vi "resonant.calculation vi_MD.vi"() -> ()   [LabVIEW 2012]
uses:
  Custom Controls/display palette control.ctl
  Custom Controls/scan mode main settings tab.ctl
  <vilib>/Utility/miscctls.llb/LVMinMaxIncTypeDef.ctl
  <vilib>/Utility/miscctls.llb/LVOutOfRangeActionTypeDef.ctl
  Custom Controls/pixel resolution enum.ctl
  Custom Controls/experiment type.ctl
  Custom Controls/advanced settings inner tab CTL.ctl
  Custom Controls/MAIN Image panel reso tab Control type def.ctl
  Custom Controls/Histogram tab reso.ctl
  GFG/GFGnumericGet.vi
  GFG/GFGfpRefGet.vi
  GFG/GFGbooleanGet.vi
  GFG/GFGDisplayRefsGet.vi
  GFG/GFGImageRefsGet.vi
  GFG/GFG library.lvlib
panel:
  out "ready for flystart?":bool
  out "Numeric Control 2":i32
  in  "String":string
  out "Source VI":string
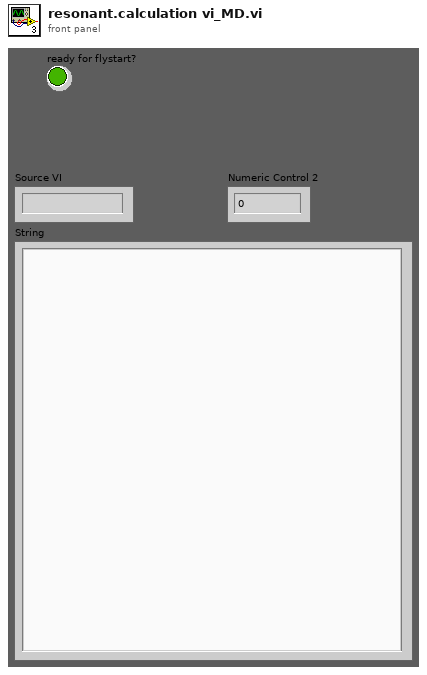
[diagram p1: front panel]
types:
  T1 = typedef "display palette control.ctl" = enum16{"standard", "high clipping red", "low clipping blue", "high and low clipping"}
  T2 = typedef "scan mode main settings tab.ctl" = enum32{"2D frame", "2D line scan", "general settings", "Z Stack", "piezo"}
  T3 = typedef "LVOutOfRangeActionTypeDef.ctl" = cluster{"Out of Range Action Minimum":u8, "Out of Range Action Maximum":u8, "Out of Range Action Increment":u8}
  T4 = typedef "LVMinMaxIncTypeDef.ctl" = cluster{"Minimum":dbl, "Maximum":dbl, "Increment":dbl}
  T5 = enum8{"Enabled", "Disabled", "Disabled and Grayed Out"}
  T6 = typedef "pixel resolution enum.ctl" = enum16{"   128 x 128", "   256 x 128", "   256 x 256", "   512 x  64", "   512 x 128", "   512 x 256", "   512 x 512", "  1024 x 512", "  1024 x 1024", "   arbitrary"}
  T7 = typedef "experiment type.ctl" = string
  T8 = enum32{"Page Enabled", "Page Disabled", "Page Disabled & Grayed"}
  T9 = typedef "advanced settings inner tab CTL.ctl" = enum32{"arb. frames", "AO", "AI", "channels", "trigger", "Zstack data"}
  T10 = typedef "MAIN Image panel reso tab Control type def.ctl" = enum32{"Channel 1", "Channel 2", "Channel 3", "Channel 4", "Channel 5", "all channels", "RGB overlay", "ROI", "arbitrary line scan"}
  T11 = typedef "Histogram tab reso.ctl" = enum32{"hist Ch 1", "hist Ch 4", "hist Ch 5", "hist Ch 3", "hist Ch 2"}
  T12 = cluster{"WaveformChartRef":refnum<vi>, "DigitalRef":refnum<vi>, "ArrayRef":refnum<vi>, "TabControlRef":refnum<vi>, "EnumRef":refnum<vi>, "RingRef":refnum<vi>, "BooleanRef":refnum<vi>, "KnobRef":refnum<vi>, "SlideRef":refnum<vi>, "PathRef":refnum<vi>, "StringRef":refnum<vi>, "ComboBox":refnum<vi>, "WaveformGraphRef":refnum<vi>}
  T13 = cluster{"Channel 1 small":refnum<vi>, "Channel 2 small":refnum<vi>, "Channel 3 small":refnum<vi>, "Channel 4 small":refnum<vi>, "Channel 1 large":refnum<vi>, "Channel 2 large":refnum<vi>, "Channel 3 large":refnum<vi>, "Channel 4 large":refnum<vi>, "RGB overlay":refnum<vi>, "ROI Image display":refnum<vi>, "arb line scan display":refnum<vi>, "Channel 5 large":refnum<vi>}
  T14 = typedef "IMAQ Image.ctl" = refnum<image>
  T15 = cluster{"Channel 1 small":T14, "Channel 2 small":T14, "Channel 3 small":T14, "Channel 4 small":T14, "Channel 1 large":T14, "Channel 2 large":T14, "Channel 3 large":T14, "Channel 4 large":T14, "RGB overlay":T14, "ROI Image display":T14, "arb line scan display":T14, "Channel 5 large":T14}
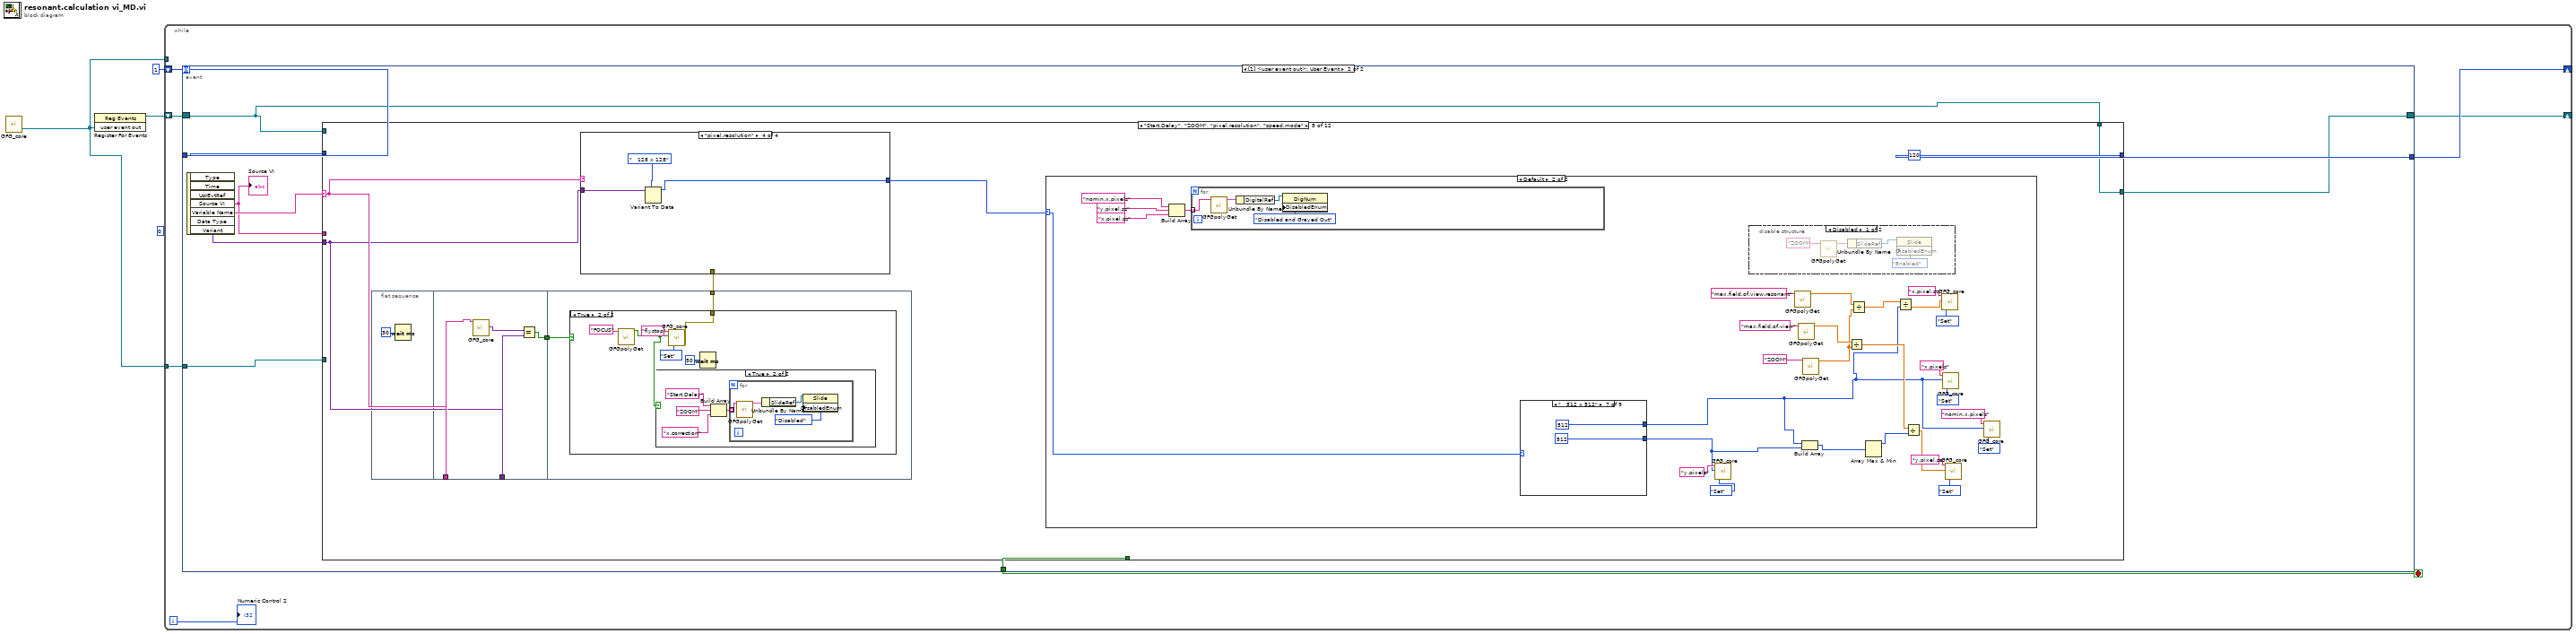
[diagram p0: block diagram]
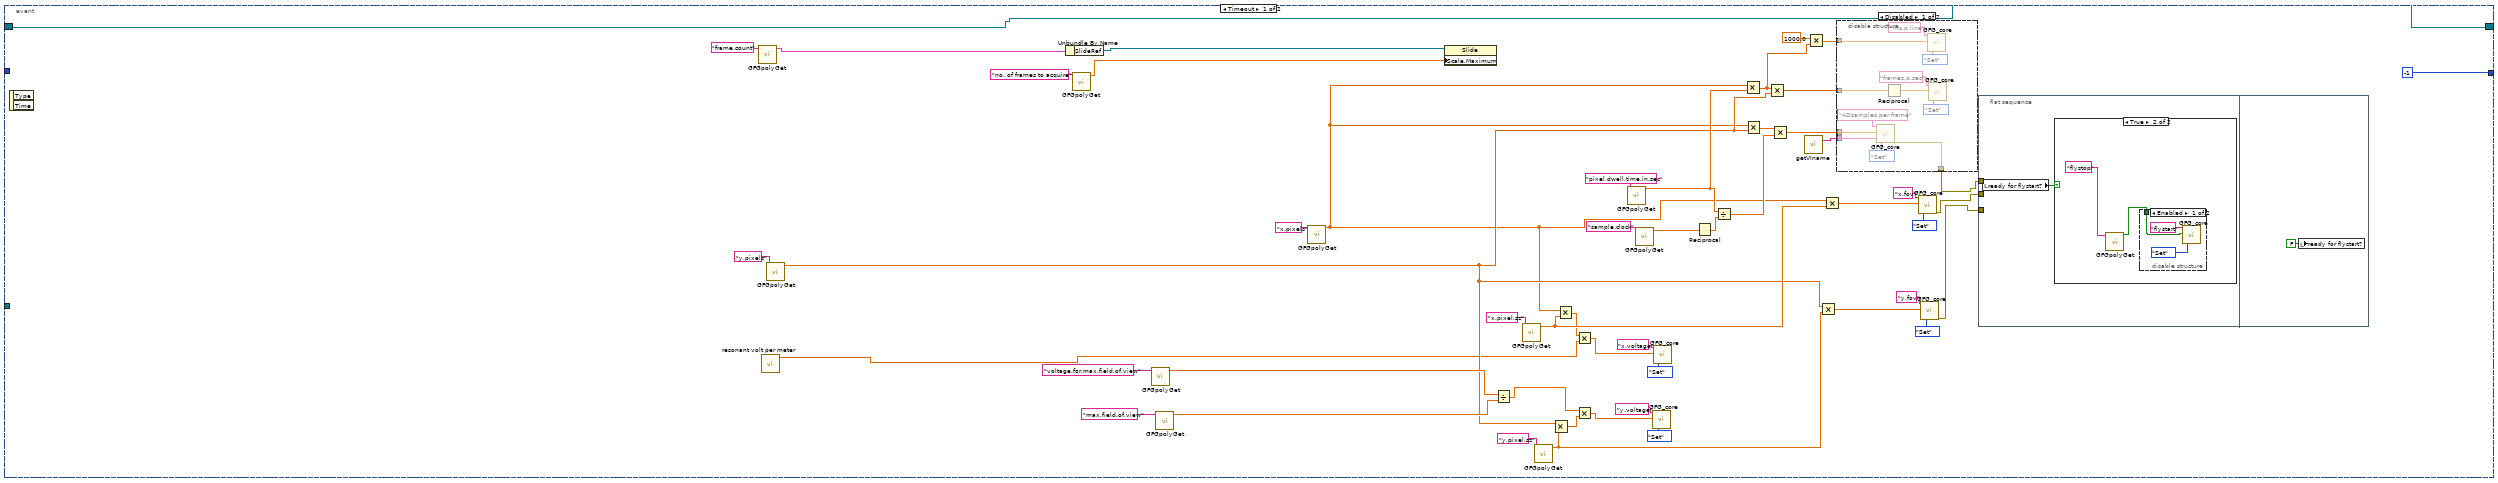
[diagram p2: hidden frame]
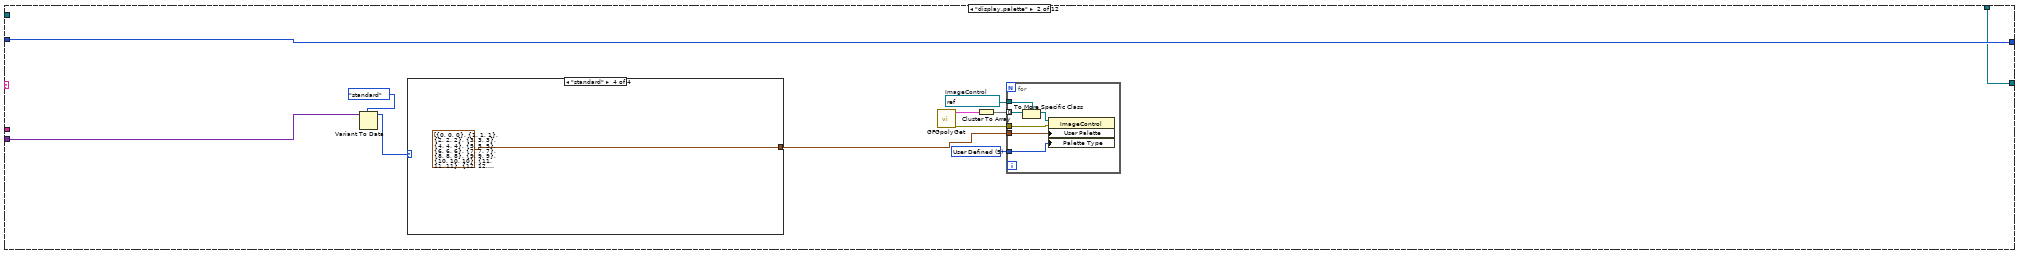
[diagram p7: hidden frame]
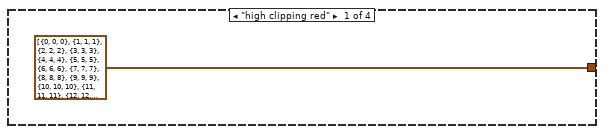
[diagram p8: hidden frame]
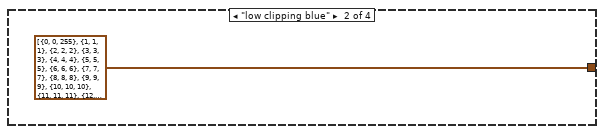
[diagram p9: hidden frame]
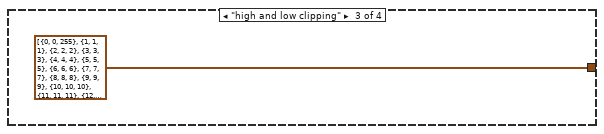
[diagram p10: hidden frame]
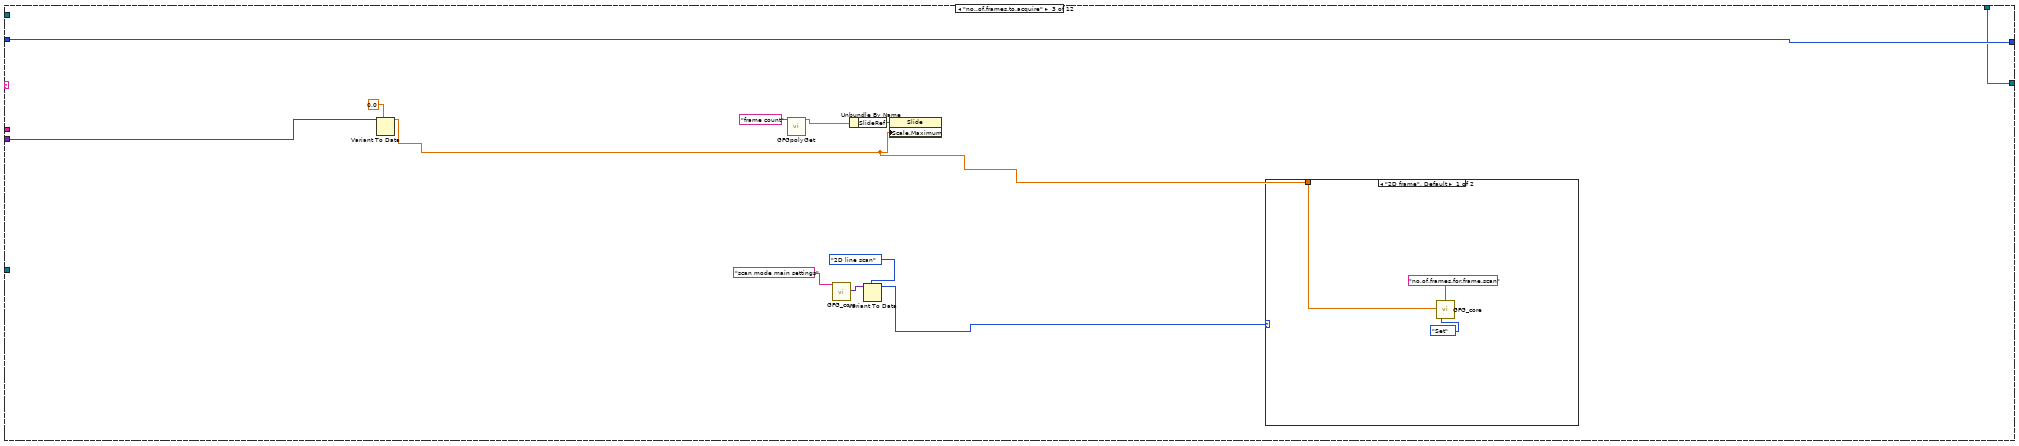
[diagram p11: hidden frame]
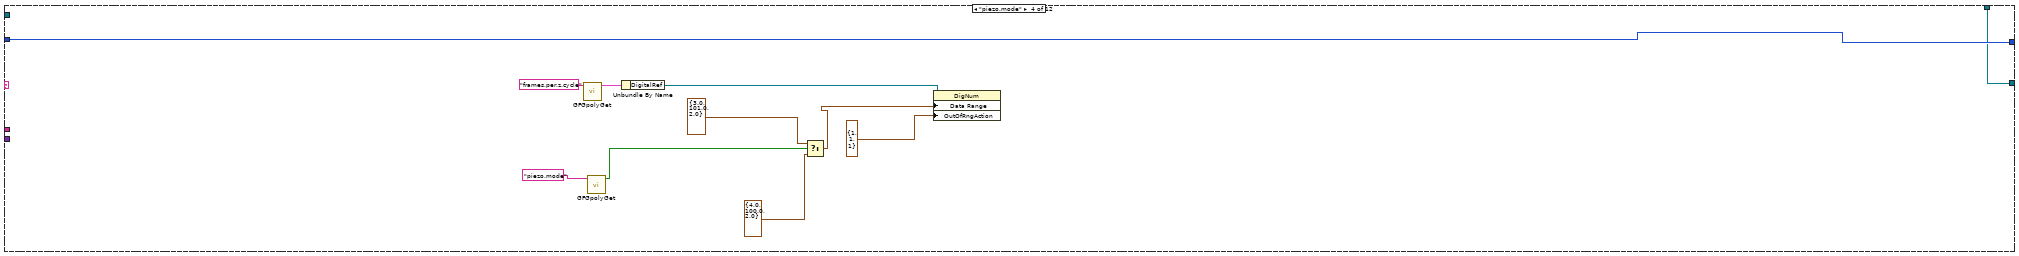
[diagram p13: hidden frame]
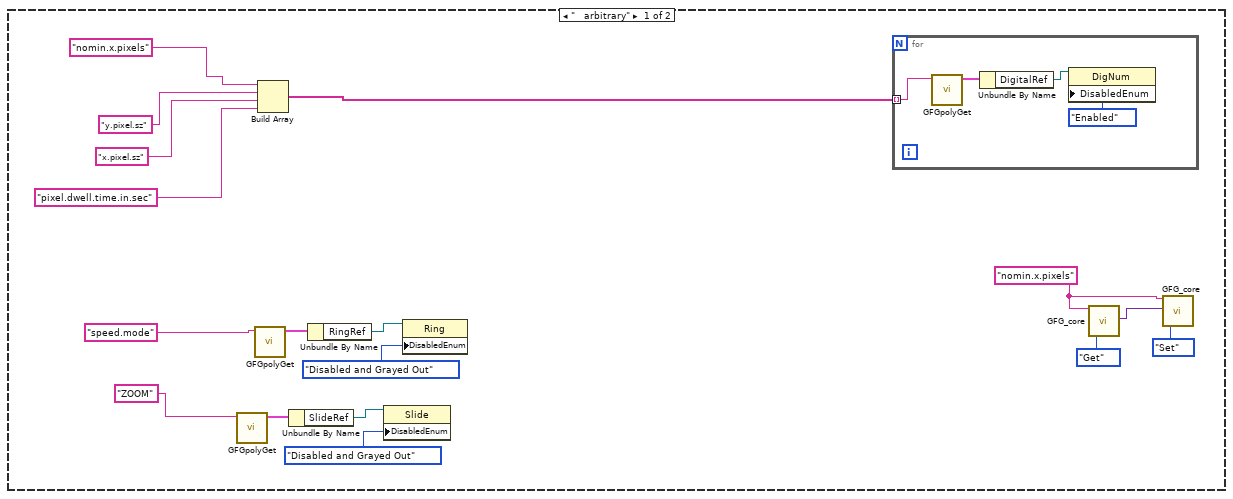
[diagram p16: hidden frame]
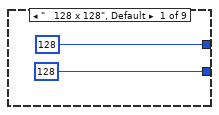
[diagram p18: hidden frame]
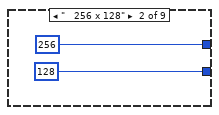
[diagram p19: hidden frame]
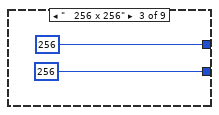
[diagram p20: hidden frame]
diagram:
  (unwired) 0
  n1 = call "GFG_core.vi"() -> ("user event out"=w1:refnum<user-event>)  [unwired: 13 in, 6 out]
  n2 = register-events(w1) -> (reference out=w3:refnum<event-registration>)  [unwired: 2 in, 1 out]
  n3 = while {
    shift-right: [w8] -> _
    shift-left: 1 -> [w7]
    tunnel: w1 -> [_]
    shift-right: [w4] -> _
    shift-left: w3 -> [w10]
    tunnel: w1 -> [w5]
    i -> [w6]
    stop <- w9 stop-if-true
    n4 = event shown="[1] <user event out>: User Event" {
      selector: w10 -> [w16 w82]
      dyn-events: [w16 w81] -> w4
      timeout: w7 -> [_ _]
      tunnel: [_ w88] -> w9
      tunnel: [-1 w86] -> w8
      tunnel: w7 -> [_ w85]
      tunnel: w5 -> [_ w83]
      event Timeout {
        n5 = event-data() -> ()  [unwired: 1 in, 2 out]
        n6 = call-poly "GFGpolyGet.vi"("Variable Name in"="frame.count") -> ("output cluster"=w20:T12)  [unwired: 9 in, 1 out]
        n7 = call "resonant volt per meter.vi"() -> ("volt/meter interpolated"=w15:dbl)  [unwired: 11 in]
        n8 = call-poly "GFGpolyGet.vi"("Variable Name in"="y.pixels") -> ("Numeric"=w22:dbl)  [unwired: 9 in, 1 out]
        n9 = Unbundle By Name(w20) -> ("SlideRef"=w19:refnum<vi>)
        n10 = call-poly "GFGpolyGet.vi"("Variable Name in"="no. of frames to acquire") -> ("Numeric"=w17:dbl)  [unwired: 9 in, 1 out]
        n11 = call-poly "GFGpolyGet.vi"("Variable Name in"="voltage.for.max.field.of.view") -> ("Numeric"=w41:dbl)  [unwired: 9 in, 1 out]
        n12 = call-poly "GFGpolyGet.vi"("Variable Name in"="max.field.of.view") -> ("Numeric"=w42:dbl)  [unwired: 9 in, 1 out]
        n13 = call-poly "GFGpolyGet.vi"("Variable Name in"="x.pixels") -> ("Numeric"=w11:dbl)  [unwired: 9 in, 1 out]
        n14 = property class="Slide"(reference=w19, "Scale.Maximum"=w17) -> ()  [unwired: 1 in, 2 out]
        n15 = Divide(x=w41, y=w42) -> (x/y=w40:dbl)
        n16 = call-poly "GFGpolyGet.vi"("Variable Name in"="x.pixel.sz") -> ("Numeric"=w33:dbl)  [unwired: 9 in, 1 out]
        n17 = call-poly "GFGpolyGet.vi"("Variable Name in"="y.pixel.sz") -> ("Numeric"=w31:dbl)  [unwired: 9 in, 1 out]
        n18 = Multiply(x=w22, y=w31) -> (x*y=w30:dbl)
        n19 = Multiply(x=w11, y=w33) -> (x*y=w32:dbl)
        n20 = Multiply(x=w32, y=w15) -> (x*y=w35:dbl)
        n21 = Multiply(x=w40, y=w30) -> (x*y=w34:dbl)
        n22 = call-poly "GFGpolyGet.vi"("Variable Name in"="pixel.dwell.time.in.sec") -> ("Numeric"=w26:dbl)  [unwired: 9 in, 1 out]
        n23 = call-poly "GFGpolyGet.vi"("Variable Name in"="sample.clock") -> ("Numeric"=w29:dbl)  [unwired: 9 in, 1 out]
        n24 = call "GFG_core.vi"("Variable Name in"="y.voltage", "Variant in"=w34, "Action"=enum16{"Init", "Set", "Get"}."Set") -> ()  [unwired: 10 in, 7 out]
        n25 = call "GFG_core.vi"("Variable Name in"="x.voltage", "Variant in"=w35, "Action"=enum16{"Init", "Set", "Get"}."Set") -> ()  [unwired: 10 in, 7 out]
        n26 = Reciprocal(x=w29) -> (1/x=w49:dbl)
        n27 = Divide(x=w26, y=w49) -> (x/y=w47:dbl)
        n28 = Multiply(x=w11, y=w26) -> (x*y=w25:dbl)
        n29 = Multiply(x=w11, y=w22) -> (x*y=w28:dbl)
        n30 = Multiply(x=w25, y=w22) -> (x*y=w27:dbl)
        n31 = Multiply(x=w28, y=w47) -> (x*y=w60:dbl)
        n32 = call "getVIname.vi"() -> ("VI name"=w59:string)  [unwired: 19 in]
        n33 = Multiply(x=1000.0, y=w25) -> (x*y=w23:dbl)
        n34 = Multiply(x=w22, y=w31) -> (x*y=w51:dbl)
        n35 = Multiply(x=w11, y=w33) -> (x*y=w54:dbl)
        n36 = disable-structure shown="Disabled" {
          disable-tunnel: w60 -> [w79 _]
          disable-tunnel: w59 -> [w77 _]
          disable-tunnel: [w76 _] -> w14
          disable-tunnel: w27 -> [w71 _]
          disable-tunnel: w23 -> [w69 _]
          frame Disabled {
            n37 = call "GFG_core.vi"("Variable Name in"="ADsamples.per.frame", "Variant in"=w79, "Source VI"=w77, "Action"=enum16{"Init", "Set", "Get"}."Set") -> ("error out"=w76:errorcluster)  [unwired: 9 in, 6 out]
            n38 = Reciprocal(x=w71) -> (1/x=w70:dbl)
            n39 = call "GFG_core.vi"("Variable Name in"="ms.p.line", "Variant in"=w69, "Action"=enum16{"Init", "Set", "Get"}."Set") -> ()  [unwired: 10 in, 7 out]
            n40 = call "GFG_core.vi"("Variable Name in"="frames.p.sec", "Variant in"=w70, "Action"=enum16{"Init", "Set", "Get"}."Set") -> ()  [unwired: 10 in, 7 out]
          }
          frame Enabled {
          }
        }
        n41 = call "GFG_core.vi"("Variable Name in"="x.fov", "Variant in"=w54, "Action"=enum16{"Init", "Set", "Get"}."Set") -> ("error out"=w13:errorcluster)  [unwired: 10 in, 6 out]
        n42 = call "GFG_core.vi"("Variable Name in"="y.fov", "Variant in"=w51, "Action"=enum16{"Init", "Set", "Get"}."Set") -> ("error out"=w12:errorcluster)  [unwired: 10 in, 6 out]
        n43 = flat-sequence {
          tunnel: w14 -> [_]
          tunnel: w13 -> [_]
          tunnel: w12 -> [_]
          frame #0 {
            n44 = local read "ready for flystart?"() -> (w62:bool)
            n45 = case shown="True" w62 {
              frame False {
              }
              frame True {
                n46 = call-poly "GFGpolyGet.vi"("Variable Name in"="flystop") -> ("Boolean"=w63:bool)  [unwired: 10 in]
                n47 = disable-structure shown="Enabled" {
                  disable-tunnel: w63 -> [w65 _]
                  frame Enabled {
                    n48 = call "GFG_core.vi"("Variable Name in"="flystart", "Variant in"=w65, "Action"=enum16{"Init", "Set", "Get"}."Set") -> ()  [unwired: 10 in, 7 out]
                  }
                  frame Disabled {
                  }
                }
              }
            }
          }
          frame #1 {
            n49 = local write "ready for flystart?"(FALSE ("ready for flystart?")) -> ()
          }
        }
      }
      event User Event {
        n50 = event-data() -> ("Source VI"=w84:string, "Variable Name"=w89:string, "Variant"=w87:variant)  [unwired: 1 in, 4 out]
        "Source VI" <- w84
        n51 = case shown="\"Start.Delay\", \"ZOOM\", \"pixel.resolution\", \"speed.mode\"" w89 {
          selector: w89 -> [_ _ _ _ w142 _ _ _ w342 _ _ _]
          tunnel: [_ _ _ _ _ _ _ _ _ _ _ TRUE] -> w88
          tunnel: w87 -> [_ w102 w121 _ w141 _ _ w296 _ w369 w399 _]
          tunnel: [w91 w99 w119 w138 120 w275 w283 w292 150 w366 w400 w402] -> w86
          tunnel: w85 -> [w91 w99 w119 w138 _ w275 w283 w293 _ w367 w400 w402]
          tunnel: w84 -> [_ _ _ _ _ _ _ _ _ _ _ _]
          tunnel: w82 -> [_ _ _ _ _ w274 _ _ _ _ _ _]
          tunnel: w83 -> [_ _ _ _ _ _ _ _ _ _ _ _]
          tunnel: [w90 w92 w113 w128 w143 w274 w284 w291 w343 w361 w380 w401] -> w81
          tunnel: w82 -> [w90 w92 w113 w128 w143 _ w284 w291 w343 w361 w380 w401]
          frame "False", Default {
          }
          frame "display.palette" {
            w94 = u32 5 items=["Grayscale", "Binary", "Gradient", "Rainbow", "Temperature", "User Defined"] ("Palette:Palette Type")
            w96 = refnum<vi> refnum  # ImageControl
            n52 = Variant To Data(type=display_palette_control."standard" ("display palette"), Variant=w102) -> (data=w100:T1)  [unwired: 1 in, 1 out]
            n53 = case shown="\"standard\"" w100 {
              tunnel: [cluster{"Red":u8, "Green":u8, "Blue":u8}[] [{"Red"=0, "Green"=0, "Blue"=0}, {"Red"=1, "Green"=1, "Blue"=1}, {"Red"=2, "Green"=2, "Blue"=2}, {"Red"=3, "Green"=3, "Blue"=3}, {"Red"=4, "Green"=4, "Blue"=4}, {"Red"=5, "Green"=5, "Blue"=5}, {"Red"=6, "Green"=6, "Blue"=6}, {"Red"=7, "Green"=7, "Blue"=7}, {"Red"=8, "Green"=8, "Blue"=8}, {"Red"=9, "Green"=9, "Blue"=9}, {"Red"=10, "Green"=10, "Blue"=10}, {"Red"=11, "Green"=11, "Blue"=11}, {"Red"=12, "Green"=12, "Blue"=12}, {"Red"=13, "Green"=13, "Blue"=13}, {"Red"=14, "Green"=14, "Blue"=14}, {"Red"=15, "Green"=15, "Blue"=15}, {"Red"=16, "Green"=16, "Blue"=16}, {"Red"=17, "Green"=17, "Blue"=17}, {"Red"=18, "Green"=18, "Blue"=18}, {"Red"=19, "Green"=19, "Blue"=19}, {"Red"=20, "Green"=20, "Blue"=20}, {"Red"=21, "Green"=21, "Blue"=21}, {"Red"=22, "Green"=22, "Blue"=22}, {"Red"=23, "Green"=23, "Blue"=23}, {"Red"=24, "Green"=24, "Blue"=24}, {"Red"=25, "Green"=25, "Blue"=25}, {"Red"=26, "Green"=26, "Blue"=26}, {"Red"=27, "Green"=27, "Blue"=27}, {"Red"=28, "Green"=28, "Blue"=28}, {"Red"=29, "Green"=29, "Blue"=29}, {"Red"=30, "Green"=30, "Blue"=30}, {"Red"=31, "Green"=31, "Blue"=31}, {"Red"=32, "Green"=32, "Blue"=32}, {"Red"=33, "Green"=33, "Blue"=33}, {"Red"=34, "Green"=34, "Blue"=34}, {"Red"=35, "Green"=35, "Blue"=35}, {"Red"=36, "Green"=36, "Blue"=36}, {"Red"=37, "Green"=37, "Blue"=37}, {"Red"=38, "Green"=38, "Blue"=38}, {"Red"=39, "Green"=39, "Blue"=39}, {"Red"=40, "Green"=40, "Blue"=40}, {"Red"=41, "Green"=41, "Blue"=41}, {"Red"=42, "Green"=42, "Blue"=42}, {"Red"=43, "Green"=43, "Blue"=43}, {"Red"=44, "Green"=44, "Blue"=44}, {"Red"=45, "Green"=45, "Blue"=45}, {"Red"=46, "Green"=46, "Blue"=46}, {"Red"=47, "Green"=47, "Blue"=47}, {"Red"=48, "Green"=48, "Blue"=48}, {"Red"=49, "Green"=49, "Blue"=49}, {"Red"=50, "Green"=50, "Blue"=50}, {"Red"=51, "Green"=51, "Blue"=51}, {"Red"=52, "Green"=52, "Blue"=52}, {"Red"=53, "Green"=53, "Blue"=53}, {"Red"=54, "Green"=54, "Blue"=54}, {"Red"=55, "Green"=55, "Blue"=55}, {"Red"=56, "Green"=56, "Blue"=56}, {"Red"=57, "Green"=57, "Blue"=57}, {"Red"=58, "Green"=58, "Blue"=58}, {"Red"=59, "Green"=59, "Blue"=59}, {"Red"=60, "Green"=60, "Blue"=60}, {"Red"=61, "Green"=61, "Blue"=61}, {"Red"=62, "Green"=62, "Blue"=62}, {"Red"=63, "Green"=63, "Blue"=63}, {"Red"=64, "Green"=64, "Blue"=64}, {"Red"=65, "Green"=65, "Blue"=65}, {"Red"=66, "Green"=66, "Blue"=66}, {"Red"=67, "Green"=67, "Blue"=67}, {"Red"=68, "Green"=68, "Blue"=68}, {"Red"=69, "Green"=69, "Blue"=69}, {"Red"=70, "Green"=70, "Blue"=70}, {"Red"=71, "Green"=71, "Blue"=71}, {"Red"=72, "Green"=72, "Blue"=72}, {"Red"=73, "Green"=73, "Blue"=73}, {"Red"=74, "Green"=74, "Blue"=74}, {"Red"=75, "Green"=75, "Blue"=75}, {"Red"=76, "Green"=76, "Blue"=76}, {"Red"=77, "Green"=77, "Blue"=77}, {"Red"=78, "Green"=78, "Blue"=78}, {"Red"=79, "Green"=79, "Blue"=79}, {"Red"=80, "Green"=80, "Blue"=80}, {"Red"=81, "Green"=81, "Blue"=81}, {"Red"=82, "Green"=82, "Blue"=82}, {"Red"=83, "Green"=83, "Blue"=83}, {"Red"=84, "Green"=84, "Blue"=84}, {"Red"=85, "Green"=85, "Blue"=85}, {"Red"=86, "Green"=86, "Blue"=86}, {"Red"=87, "Green"=87, "Blue"=87}, {"Red"=88, "Green"=88, "Blue"=88}, {"Red"=89, "Green"=89, "Blue"=89}, {"Red"=90, "Green"=90, "Blue"=90}, {"Red"=91, "Green"=91, "Blue"=91}, {"Red"=92, "Green"=92, "Blue"=92}, {"Red"=93, "Green"=93, "Blue"=93}, {"Red"=94, "Green"=94, "Blue"=94}, {"Red"=95, "Green"=95, "Blue"=95}, {"Red"=96, "Green"=96, "Blue"=96}, {"Red"=97, "Green"=97, "Blue"=97}, {"Red"=98, "Green"=98, "Blue"=98}, {"Red"=99, "Green"=99, "Blue"=99}, {"Red"=100, "Green"=100, "Blue"=100}, {"Red"=101, "Green"=101, "Blue"=101}, {"Red"=102, "Green"=102, "Blue"=102}, {"Red"=103, "Green"=103, "Blue"=103}, {"Red"=104, "Green"=104, "Blue"=104}, {"Red"=105, "Green"=105, "Blue"=105}, {"Red"=106, "Green"=106, "Blue"=106}, {"Red"=107, "Green"=107, "Blue"=107}, {"Red"=108, "Green"=108, "Blue"=108}, {"Red"=109, "Green"=109, "Blue"=109}, {"Red"=110, "Green"=110, "Blue"=110}, {"Red"=111, "Green"=111, "Blue"=111}, {"Red"=112, "Green"=112, "Blue"=112}, {"Red"=113, "Green"=113, "Blue"=113}, {"Red"=114, "Green"=114, "Blue"=114}, {"Red"=115, "Green"=115, "Blue"=115}, {"Red"=116, "Green"=116, "Blue"=116}, {"Red"=117, "Green"=117, "Blue"=117}, {"Red"=118, "Green"=118, "Blue"=118}, {"Red"=119, "Green"=119, "Blue"=119}, {"Red"=120, "Green"=120, "Blue"=120}, {"Red"=121, "Green"=121, "Blue"=121}, {"Red"=122, "Green"=122, "Blue"=122}, {"Red"=123, "Green"=123, "Blue"=123}, {"Red"=124, "Green"=124, "Blue"=124}, {"Red"=125, "Green"=125, "Blue"=125}, {"Red"=126, "Green"=126, "Blue"=126}, {"Red"=127, "Green"=127, "Blue"=127}, {"Red"=128, "Green"=128, "Blue"=128}, {"Red"=129, "Green"=129, "Blue"=129}, {"Red"=130, "Green"=130, "Blue"=130}, {"Red"=131, "Green"=131, "Blue"=131}, {"Red"=132, "Green"=132, "Blue"=132}, {"Red"=133, "Green"=133, "Blue"=133}, {"Red"=134, "Green"=134, "Blue"=134}, {"Red"=135, "Green"=135, "Blue"=135}, {"Red"=136, "Green"=136, "Blue"=136}, {"Red"=137, "Green"=137, "Blue"=137}, {"Red"=138, "Green"=138, "Blue"=138}, {"Red"=139, "Green"=139, "Blue"=139}, {"Red"=140, "Green"=140, "Blue"=140}, {"Red"=141, "Green"=141, "Blue"=141}, {"Red"=142, "Green"=142, "Blue"=142}, {"Red"=143, "Green"=143, "Blue"=143}, {"Red"=144, "Green"=144, "Blue"=144}, {"Red"=145, "Green"=145, "Blue"=145}, {"Red"=146, "Green"=146, "Blue"=146}, {"Red"=147, "Green"=147, "Blue"=147}, {"Red"=148, "Green"=148, "Blue"=148}, {"Red"=149, "Green"=149, "Blue"=149}, {"Red"=150, "Green"=150, "Blue"=150}, {"Red"=151, "Green"=151, "Blue"=151}, {"Red"=152, "Green"=152, "Blue"=152}, {"Red"=153, "Green"=153, "Blue"=153}, {"Red"=154, "Green"=154, "Blue"=154}, {"Red"=155, "Green"=155, "Blue"=155}, {"Red"=156, "Green"=156, "Blue"=156}, {"Red"=157, "Green"=157, "Blue"=157}, {"Red"=158, "Green"=158, "Blue"=158}, {"Red"=159, "Green"=159, "Blue"=159}, {"Red"=160, "Green"=160, "Blue"=160}, {"Red"=161, "Green"=161, "Blue"=161}, {"Red"=162, "Green"=162, "Blue"=162}, {"Red"=163, "Green"=163, "Blue"=163}, {"Red"=164, "Green"=164, "Blue"=164}, {"Red"=165, "Green"=165, "Blue"=165}, {"Red"=166, "Green"=166, "Blue"=166}, {"Red"=167, "Green"=167, "Blue"=167}, {"Red"=168, "Green"=168, "Blue"=168}, {"Red"=169, "Green"=169, "Blue"=169}, {"Red"=170, "Green"=170, "Blue"=170}, {"Red"=171, "Green"=171, "Blue"=171}, {"Red"=172, "Green"=172, "Blue"=172}, {"Red"=173, "Green"=173, "Blue"=173}, {"Red"=174, "Green"=174, "Blue"=174}, {"Red"=175, "Green"=175, "Blue"=175}, {"Red"=176, "Green"=176, "Blue"=176}, {"Red"=177, "Green"=177, "Blue"=177}, {"Red"=178, "Green"=178, "Blue"=178}, {"Red"=179, "Green"=179, "Blue"=179}, {"Red"=180, "Green"=180, "Blue"=180}, {"Red"=181, "Green"=181, "Blue"=181}, {"Red"=182, "Green"=182, "Blue"=182}, {"Red"=183, "Green"=183, "Blue"=183}, {"Red"=184, "Green"=184, "Blue"=184}, {"Red"=185, "Green"=185, "Blue"=185}, {"Red"=186, "Green"=186, "Blue"=186}, {"Red"=187, "Green"=187, "Blue"=187}, {"Red"=188, "Green"=188, "Blue"=188}, {"Red"=189, "Green"=189, "Blue"=189}, {"Red"=190, "Green"=190, "Blue"=190}, {"Red"=191, "Green"=191, "Blue"=191}, {"Red"=192, "Green"=192, "Blue"=192}, {"Red"=193, "Green"=193, "Blue"=193}, {"Red"=194, "Green"=194, "Blue"=194}, {"Red"=195, "Green"=195, "Blue"=195}, {"Red"=196, "Green"=196, "Blue"=196}, {"Red"=197, "Green"=197, "Blue"=197}, {"Red"=198, "Green"=198, "Blue"=198}, {"Red"=199, "Green"=199, "Blue"=199}, {"Red"=200, "Green"=200, "Blue"=200}, {"Red"=201, "Green"=201, "Blue"=201}, {"Red"=202, "Green"=202, "Blue"=202}, {"Red"=203, "Green"=203, "Blue"=203}, {"Red"=204, "Green"=204, "Blue"=204}, {"Red"=205, "Green"=205, "Blue"=205}, {"Red"=206, "Green"=206, "Blue"=206}, {"Red"=207, "Green"=207, "Blue"=207}, {"Red"=208, "Green"=208, "Blue"=208}, {"Red"=209, "Green"=209, "Blue"=209}, {"Red"=210, "Green"=210, "Blue"=210}, {"Red"=211, "Green"=211, "Blue"=211}, {"Red"=212, "Green"=212, "Blue"=212}, {"Red"=213, "Green"=213, "Blue"=213}, {"Red"=214, "Green"=214, "Blue"=214}, {"Red"=215, "Green"=215, "Blue"=215}, {"Red"=216, "Green"=216, "Blue"=216}, {"Red"=217, "Green"=217, "Blue"=217}, {"Red"=218, "Green"=218, "Blue"=218}, {"Red"=219, "Green"=219, "Blue"=219}, {"Red"=220, "Green"=220, "Blue"=220}, {"Red"=221, "Green"=221, "Blue"=221}, {"Red"=222, "Green"=222, "Blue"=222}, {"Red"=223, "Green"=223, "Blue"=223}, {"Red"=224, "Green"=224, "Blue"=224}, {"Red"=225, "Green"=225, "Blue"=225}, {"Red"=226, "Green"=226, "Blue"=226}, {"Red"=227, "Green"=227, "Blue"=227}, {"Red"=228, "Green"=228, "Blue"=228}, {"Red"=229, "Green"=229, "Blue"=229}, {"Red"=230, "Green"=230, "Blue"=230}, {"Red"=231, "Green"=231, "Blue"=231}, {"Red"=232, "Green"=232, "Blue"=232}, {"Red"=233, "Green"=233, "Blue"=233}, {"Red"=234, "Green"=234, "Blue"=234}, {"Red"=235, "Green"=235, "Blue"=235}, {"Red"=236, "Green"=236, "Blue"=236}, {"Red"=237, "Green"=237, "Blue"=237}, {"Red"=238, "Green"=238, "Blue"=238}, {"Red"=239, "Green"=239, "Blue"=239}, {"Red"=240, "Green"=240, "Blue"=240}, {"Red"=241, "Green"=241, "Blue"=241}, {"Red"=242, "Green"=242, "Blue"=242}, {"Red"=243, "Green"=243, "Blue"=243}, {"Red"=244, "Green"=244, "Blue"=244}, {"Red"=245, "Green"=245, "Blue"=245}, {"Red"=246, "Green"=246, "Blue"=246}, {"Red"=247, "Green"=247, "Blue"=247}, {"Red"=248, "Green"=248, "Blue"=248}, {"Red"=249, "Green"=249, "Blue"=249}, {"Red"=250, "Green"=250, "Blue"=250}, {"Red"=251, "Green"=251, "Blue"=251}, {"Red"=252, "Green"=252, "Blue"=252}, {"Red"=253, "Green"=253, "Blue"=253}, {"Red"=254, "Green"=254, "Blue"=254}, {"Red"=255, "Green"=0, "Blue"=0}] ("Color Palette") cluster{"Red":u8, "Green":u8, "Blue":u8}[] [{"Red"=0, "Green"=0, "Blue"=255}, {"Red"=1, "Green"=1, "Blue"=1}, {"Red"=2, "Green"=2, "Blue"=2}, {"Red"=3, "Green"=3, "Blue"=3}, {"Red"=4, "Green"=4, "Blue"=4}, {"Red"=5, "Green"=5, "Blue"=5}, {"Red"=6, "Green"=6, "Blue"=6}, {"Red"=7, "Green"=7, "Blue"=7}, {"Red"=8, "Green"=8, "Blue"=8}, {"Red"=9, "Green"=9, "Blue"=9}, {"Red"=10, "Green"=10, "Blue"=10}, {"Red"=11, "Green"=11, "Blue"=11}, {"Red"=12, "Green"=12, "Blue"=12}, {"Red"=13, "Green"=13, "Blue"=13}, {"Red"=14, "Green"=14, "Blue"=14}, {"Red"=15, "Green"=15, "Blue"=15}, {"Red"=16, "Green"=16, "Blue"=16}, {"Red"=17, "Green"=17, "Blue"=17}, {"Red"=18, "Green"=18, "Blue"=18}, {"Red"=19, "Green"=19, "Blue"=19}, {"Red"=20, "Green"=20, "Blue"=20}, {"Red"=21, "Green"=21, "Blue"=21}, {"Red"=22, "Green"=22, "Blue"=22}, {"Red"=23, "Green"=23, "Blue"=23}, {"Red"=24, "Green"=24, "Blue"=24}, {"Red"=25, "Green"=25, "Blue"=25}, {"Red"=26, "Green"=26, "Blue"=26}, {"Red"=27, "Green"=27, "Blue"=27}, {"Red"=28, "Green"=28, "Blue"=28}, {"Red"=29, "Green"=29, "Blue"=29}, {"Red"=30, "Green"=30, "Blue"=30}, {"Red"=31, "Green"=31, "Blue"=31}, {"Red"=32, "Green"=32, "Blue"=32}, {"Red"=33, "Green"=33, "Blue"=33}, {"Red"=34, "Green"=34, "Blue"=34}, {"Red"=35, "Green"=35, "Blue"=35}, {"Red"=36, "Green"=36, "Blue"=36}, {"Red"=37, "Green"=37, "Blue"=37}, {"Red"=38, "Green"=38, "Blue"=38}, {"Red"=39, "Green"=39, "Blue"=39}, {"Red"=40, "Green"=40, "Blue"=40}, {"Red"=41, "Green"=41, "Blue"=41}, {"Red"=42, "Green"=42, "Blue"=42}, {"Red"=43, "Green"=43, "Blue"=43}, {"Red"=44, "Green"=44, "Blue"=44}, {"Red"=45, "Green"=45, "Blue"=45}, {"Red"=46, "Green"=46, "Blue"=46}, {"Red"=47, "Green"=47, "Blue"=47}, {"Red"=48, "Green"=48, "Blue"=48}, {"Red"=49, "Green"=49, "Blue"=49}, {"Red"=50, "Green"=50, "Blue"=50}, {"Red"=51, "Green"=51, "Blue"=51}, {"Red"=52, "Green"=52, "Blue"=52}, {"Red"=53, "Green"=53, "Blue"=53}, {"Red"=54, "Green"=54, "Blue"=54}, {"Red"=55, "Green"=55, "Blue"=55}, {"Red"=56, "Green"=56, "Blue"=56}, {"Red"=57, "Green"=57, "Blue"=57}, {"Red"=58, "Green"=58, "Blue"=58}, {"Red"=59, "Green"=59, "Blue"=59}, {"Red"=60, "Green"=60, "Blue"=60}, {"Red"=61, "Green"=61, "Blue"=61}, {"Red"=62, "Green"=62, "Blue"=62}, {"Red"=63, "Green"=63, "Blue"=63}, {"Red"=64, "Green"=64, "Blue"=64}, {"Red"=65, "Green"=65, "Blue"=65}, {"Red"=66, "Green"=66, "Blue"=66}, {"Red"=67, "Green"=67, "Blue"=67}, {"Red"=68, "Green"=68, "Blue"=68}, {"Red"=69, "Green"=69, "Blue"=69}, {"Red"=70, "Green"=70, "Blue"=70}, {"Red"=71, "Green"=71, "Blue"=71}, {"Red"=72, "Green"=72, "Blue"=72}, {"Red"=73, "Green"=73, "Blue"=73}, {"Red"=74, "Green"=74, "Blue"=74}, {"Red"=75, "Green"=75, "Blue"=75}, {"Red"=76, "Green"=76, "Blue"=76}, {"Red"=77, "Green"=77, "Blue"=77}, {"Red"=78, "Green"=78, "Blue"=78}, {"Red"=79, "Green"=79, "Blue"=79}, {"Red"=80, "Green"=80, "Blue"=80}, {"Red"=81, "Green"=81, "Blue"=81}, {"Red"=82, "Green"=82, "Blue"=82}, {"Red"=83, "Green"=83, "Blue"=83}, {"Red"=84, "Green"=84, "Blue"=84}, {"Red"=85, "Green"=85, "Blue"=85}, {"Red"=86, "Green"=86, "Blue"=86}, {"Red"=87, "Green"=87, "Blue"=87}, {"Red"=88, "Green"=88, "Blue"=88}, {"Red"=89, "Green"=89, "Blue"=89}, {"Red"=90, "Green"=90, "Blue"=90}, {"Red"=91, "Green"=91, "Blue"=91}, {"Red"=92, "Green"=92, "Blue"=92}, {"Red"=93, "Green"=93, "Blue"=93}, {"Red"=94, "Green"=94, "Blue"=94}, {"Red"=95, "Green"=95, "Blue"=95}, {"Red"=96, "Green"=96, "Blue"=96}, {"Red"=97, "Green"=97, "Blue"=97}, {"Red"=98, "Green"=98, "Blue"=98}, {"Red"=99, "Green"=99, "Blue"=99}, {"Red"=100, "Green"=100, "Blue"=100}, {"Red"=101, "Green"=101, "Blue"=101}, {"Red"=102, "Green"=102, "Blue"=102}, {"Red"=103, "Green"=103, "Blue"=103}, {"Red"=104, "Green"=104, "Blue"=104}, {"Red"=105, "Green"=105, "Blue"=105}, {"Red"=106, "Green"=106, "Blue"=106}, {"Red"=107, "Green"=107, "Blue"=107}, {"Red"=108, "Green"=108, "Blue"=108}, {"Red"=109, "Green"=109, "Blue"=109}, {"Red"=110, "Green"=110, "Blue"=110}, {"Red"=111, "Green"=111, "Blue"=111}, {"Red"=112, "Green"=112, "Blue"=112}, {"Red"=113, "Green"=113, "Blue"=113}, {"Red"=114, "Green"=114, "Blue"=114}, {"Red"=115, "Green"=115, "Blue"=115}, {"Red"=116, "Green"=116, "Blue"=116}, {"Red"=117, "Green"=117, "Blue"=117}, {"Red"=118, "Green"=118, "Blue"=118}, {"Red"=119, "Green"=119, "Blue"=119}, {"Red"=120, "Green"=120, "Blue"=120}, {"Red"=121, "Green"=121, "Blue"=121}, {"Red"=122, "Green"=122, "Blue"=122}, {"Red"=123, "Green"=123, "Blue"=123}, {"Red"=124, "Green"=124, "Blue"=124}, {"Red"=125, "Green"=125, "Blue"=125}, {"Red"=126, "Green"=126, "Blue"=126}, {"Red"=127, "Green"=127, "Blue"=127}, {"Red"=128, "Green"=128, "Blue"=128}, {"Red"=129, "Green"=129, "Blue"=129}, {"Red"=130, "Green"=130, "Blue"=130}, {"Red"=131, "Green"=131, "Blue"=131}, {"Red"=132, "Green"=132, "Blue"=132}, {"Red"=133, "Green"=133, "Blue"=133}, {"Red"=134, "Green"=134, "Blue"=134}, {"Red"=135, "Green"=135, "Blue"=135}, {"Red"=136, "Green"=136, "Blue"=136}, {"Red"=137, "Green"=137, "Blue"=137}, {"Red"=138, "Green"=138, "Blue"=138}, {"Red"=139, "Green"=139, "Blue"=139}, {"Red"=140, "Green"=140, "Blue"=140}, {"Red"=141, "Green"=141, "Blue"=141}, {"Red"=142, "Green"=142, "Blue"=142}, {"Red"=143, "Green"=143, "Blue"=143}, {"Red"=144, "Green"=144, "Blue"=144}, {"Red"=145, "Green"=145, "Blue"=145}, {"Red"=146, "Green"=146, "Blue"=146}, {"Red"=147, "Green"=147, "Blue"=147}, {"Red"=148, "Green"=148, "Blue"=148}, {"Red"=149, "Green"=149, "Blue"=149}, {"Red"=150, "Green"=150, "Blue"=150}, {"Red"=151, "Green"=151, "Blue"=151}, {"Red"=152, "Green"=152, "Blue"=152}, {"Red"=153, "Green"=153, "Blue"=153}, {"Red"=154, "Green"=154, "Blue"=154}, {"Red"=155, "Green"=155, "Blue"=155}, {"Red"=156, "Green"=156, "Blue"=156}, {"Red"=157, "Green"=157, "Blue"=157}, {"Red"=158, "Green"=158, "Blue"=158}, {"Red"=159, "Green"=159, "Blue"=159}, {"Red"=160, "Green"=160, "Blue"=160}, {"Red"=161, "Green"=161, "Blue"=161}, {"Red"=162, "Green"=162, "Blue"=162}, {"Red"=163, "Green"=163, "Blue"=163}, {"Red"=164, "Green"=164, "Blue"=164}, {"Red"=165, "Green"=165, "Blue"=165}, {"Red"=166, "Green"=166, "Blue"=166}, {"Red"=167, "Green"=167, "Blue"=167}, {"Red"=168, "Green"=168, "Blue"=168}, {"Red"=169, "Green"=169, "Blue"=169}, {"Red"=170, "Green"=170, "Blue"=170}, {"Red"=171, "Green"=171, "Blue"=171}, {"Red"=172, "Green"=172, "Blue"=172}, {"Red"=173, "Green"=173, "Blue"=173}, {"Red"=174, "Green"=174, "Blue"=174}, {"Red"=175, "Green"=175, "Blue"=175}, {"Red"=176, "Green"=176, "Blue"=176}, {"Red"=177, "Green"=177, "Blue"=177}, {"Red"=178, "Green"=178, "Blue"=178}, {"Red"=179, "Green"=179, "Blue"=179}, {"Red"=180, "Green"=180, "Blue"=180}, {"Red"=181, "Green"=181, "Blue"=181}, {"Red"=182, "Green"=182, "Blue"=182}, {"Red"=183, "Green"=183, "Blue"=183}, {"Red"=184, "Green"=184, "Blue"=184}, {"Red"=185, "Green"=185, "Blue"=185}, {"Red"=186, "Green"=186, "Blue"=186}, {"Red"=187, "Green"=187, "Blue"=187}, {"Red"=188, "Green"=188, "Blue"=188}, {"Red"=189, "Green"=189, "Blue"=189}, {"Red"=190, "Green"=190, "Blue"=190}, {"Red"=191, "Green"=191, "Blue"=191}, {"Red"=192, "Green"=192, "Blue"=192}, {"Red"=193, "Green"=193, "Blue"=193}, {"Red"=194, "Green"=194, "Blue"=194}, {"Red"=195, "Green"=195, "Blue"=195}, {"Red"=196, "Green"=196, "Blue"=196}, {"Red"=197, "Green"=197, "Blue"=197}, {"Red"=198, "Green"=198, "Blue"=198}, {"Red"=199, "Green"=199, "Blue"=199}, {"Red"=200, "Green"=200, "Blue"=200}, {"Red"=201, "Green"=201, "Blue"=201}, {"Red"=202, "Green"=202, "Blue"=202}, {"Red"=203, "Green"=203, "Blue"=203}, {"Red"=204, "Green"=204, "Blue"=204}, {"Red"=205, "Green"=205, "Blue"=205}, {"Red"=206, "Green"=206, "Blue"=206}, {"Red"=207, "Green"=207, "Blue"=207}, {"Red"=208, "Green"=208, "Blue"=208}, {"Red"=209, "Green"=209, "Blue"=209}, {"Red"=210, "Green"=210, "Blue"=210}, {"Red"=211, "Green"=211, "Blue"=211}, {"Red"=212, "Green"=212, "Blue"=212}, {"Red"=213, "Green"=213, "Blue"=213}, {"Red"=214, "Green"=214, "Blue"=214}, {"Red"=215, "Green"=215, "Blue"=215}, {"Red"=216, "Green"=216, "Blue"=216}, {"Red"=217, "Green"=217, "Blue"=217}, {"Red"=218, "Green"=218, "Blue"=218}, {"Red"=219, "Green"=219, "Blue"=219}, {"Red"=220, "Green"=220, "Blue"=220}, {"Red"=221, "Green"=221, "Blue"=221}, {"Red"=222, "Green"=222, "Blue"=222}, {"Red"=223, "Green"=223, "Blue"=223}, {"Red"=224, "Green"=224, "Blue"=224}, {"Red"=225, "Green"=225, "Blue"=225}, {"Red"=226, "Green"=226, "Blue"=226}, {"Red"=227, "Green"=227, "Blue"=227}, {"Red"=228, "Green"=228, "Blue"=228}, {"Red"=229, "Green"=229, "Blue"=229}, {"Red"=230, "Green"=230, "Blue"=230}, {"Red"=231, "Green"=231, "Blue"=231}, {"Red"=232, "Green"=232, "Blue"=232}, {"Red"=233, "Green"=233, "Blue"=233}, {"Red"=234, "Green"=234, "Blue"=234}, {"Red"=235, "Green"=235, "Blue"=235}, {"Red"=236, "Green"=236, "Blue"=236}, {"Red"=237, "Green"=237, "Blue"=237}, {"Red"=238, "Green"=238, "Blue"=238}, {"Red"=239, "Green"=239, "Blue"=239}, {"Red"=240, "Green"=240, "Blue"=240}, {"Red"=241, "Green"=241, "Blue"=241}, {"Red"=242, "Green"=242, "Blue"=242}, {"Red"=243, "Green"=243, "Blue"=243}, {"Red"=244, "Green"=244, "Blue"=244}, {"Red"=245, "Green"=245, "Blue"=245}, {"Red"=246, "Green"=246, "Blue"=246}, {"Red"=247, "Green"=247, "Blue"=247}, {"Red"=248, "Green"=248, "Blue"=248}, {"Red"=249, "Green"=249, "Blue"=249}, {"Red"=250, "Green"=250, "Blue"=250}, {"Red"=251, "Green"=251, "Blue"=251}, {"Red"=252, "Green"=252, "Blue"=252}, {"Red"=253, "Green"=253, "Blue"=253}, {"Red"=254, "Green"=254, "Blue"=254}, {"Red"=255, "Green"=255, "Blue"=255}] ("Color Palette") cluster{"Red":u8, "Green":u8, "Blue":u8}[] [{"Red"=0, "Green"=0, "Blue"=255}, {"Red"=1, "Green"=1, "Blue"=1}, {"Red"=2, "Green"=2, "Blue"=2}, {"Red"=3, "Green"=3, "Blue"=3}, {"Red"=4, "Green"=4, "Blue"=4}, {"Red"=5, "Green"=5, "Blue"=5}, {"Red"=6, "Green"=6, "Blue"=6}, {"Red"=7, "Green"=7, "Blue"=7}, {"Red"=8, "Green"=8, "Blue"=8}, {"Red"=9, "Green"=9, "Blue"=9}, {"Red"=10, "Green"=10, "Blue"=10}, {"Red"=11, "Green"=11, "Blue"=11}, {"Red"=12, "Green"=12, "Blue"=12}, {"Red"=13, "Green"=13, "Blue"=13}, {"Red"=14, "Green"=14, "Blue"=14}, {"Red"=15, "Green"=15, "Blue"=15}, {"Red"=16, "Green"=16, "Blue"=16}, {"Red"=17, "Green"=17, "Blue"=17}, {"Red"=18, "Green"=18, "Blue"=18}, {"Red"=19, "Green"=19, "Blue"=19}, {"Red"=20, "Green"=20, "Blue"=20}, {"Red"=21, "Green"=21, "Blue"=21}, {"Red"=22, "Green"=22, "Blue"=22}, {"Red"=23, "Green"=23, "Blue"=23}, {"Red"=24, "Green"=24, "Blue"=24}, {"Red"=25, "Green"=25, "Blue"=25}, {"Red"=26, "Green"=26, "Blue"=26}, {"Red"=27, "Green"=27, "Blue"=27}, {"Red"=28, "Green"=28, "Blue"=28}, {"Red"=29, "Green"=29, "Blue"=29}, {"Red"=30, "Green"=30, "Blue"=30}, {"Red"=31, "Green"=31, "Blue"=31}, {"Red"=32, "Green"=32, "Blue"=32}, {"Red"=33, "Green"=33, "Blue"=33}, {"Red"=34, "Green"=34, "Blue"=34}, {"Red"=35, "Green"=35, "Blue"=35}, {"Red"=36, "Green"=36, "Blue"=36}, {"Red"=37, "Green"=37, "Blue"=37}, {"Red"=38, "Green"=38, "Blue"=38}, {"Red"=39, "Green"=39, "Blue"=39}, {"Red"=40, "Green"=40, "Blue"=40}, {"Red"=41, "Green"=41, "Blue"=41}, {"Red"=42, "Green"=42, "Blue"=42}, {"Red"=43, "Green"=43, "Blue"=43}, {"Red"=44, "Green"=44, "Blue"=44}, {"Red"=45, "Green"=45, "Blue"=45}, {"Red"=46, "Green"=46, "Blue"=46}, {"Red"=47, "Green"=47, "Blue"=47}, {"Red"=48, "Green"=48, "Blue"=48}, {"Red"=49, "Green"=49, "Blue"=49}, {"Red"=50, "Green"=50, "Blue"=50}, {"Red"=51, "Green"=51, "Blue"=51}, {"Red"=52, "Green"=52, "Blue"=52}, {"Red"=53, "Green"=53, "Blue"=53}, {"Red"=54, "Green"=54, "Blue"=54}, {"Red"=55, "Green"=55, "Blue"=55}, {"Red"=56, "Green"=56, "Blue"=56}, {"Red"=57, "Green"=57, "Blue"=57}, {"Red"=58, "Green"=58, "Blue"=58}, {"Red"=59, "Green"=59, "Blue"=59}, {"Red"=60, "Green"=60, "Blue"=60}, {"Red"=61, "Green"=61, "Blue"=61}, {"Red"=62, "Green"=62, "Blue"=62}, {"Red"=63, "Green"=63, "Blue"=63}, {"Red"=64, "Green"=64, "Blue"=64}, {"Red"=65, "Green"=65, "Blue"=65}, {"Red"=66, "Green"=66, "Blue"=66}, {"Red"=67, "Green"=67, "Blue"=67}, {"Red"=68, "Green"=68, "Blue"=68}, {"Red"=69, "Green"=69, "Blue"=69}, {"Red"=70, "Green"=70, "Blue"=70}, {"Red"=71, "Green"=71, "Blue"=71}, {"Red"=72, "Green"=72, "Blue"=72}, {"Red"=73, "Green"=73, "Blue"=73}, {"Red"=74, "Green"=74, "Blue"=74}, {"Red"=75, "Green"=75, "Blue"=75}, {"Red"=76, "Green"=76, "Blue"=76}, {"Red"=77, "Green"=77, "Blue"=77}, {"Red"=78, "Green"=78, "Blue"=78}, {"Red"=79, "Green"=79, "Blue"=79}, {"Red"=80, "Green"=80, "Blue"=80}, {"Red"=81, "Green"=81, "Blue"=81}, {"Red"=82, "Green"=82, "Blue"=82}, {"Red"=83, "Green"=83, "Blue"=83}, {"Red"=84, "Green"=84, "Blue"=84}, {"Red"=85, "Green"=85, "Blue"=85}, {"Red"=86, "Green"=86, "Blue"=86}, {"Red"=87, "Green"=87, "Blue"=87}, {"Red"=88, "Green"=88, "Blue"=88}, {"Red"=89, "Green"=89, "Blue"=89}, {"Red"=90, "Green"=90, "Blue"=90}, {"Red"=91, "Green"=91, "Blue"=91}, {"Red"=92, "Green"=92, "Blue"=92}, {"Red"=93, "Green"=93, "Blue"=93}, {"Red"=94, "Green"=94, "Blue"=94}, {"Red"=95, "Green"=95, "Blue"=95}, {"Red"=96, "Green"=96, "Blue"=96}, {"Red"=97, "Green"=97, "Blue"=97}, {"Red"=98, "Green"=98, "Blue"=98}, {"Red"=99, "Green"=99, "Blue"=99}, {"Red"=100, "Green"=100, "Blue"=100}, {"Red"=101, "Green"=101, "Blue"=101}, {"Red"=102, "Green"=102, "Blue"=102}, {"Red"=103, "Green"=103, "Blue"=103}, {"Red"=104, "Green"=104, "Blue"=104}, {"Red"=105, "Green"=105, "Blue"=105}, {"Red"=106, "Green"=106, "Blue"=106}, {"Red"=107, "Green"=107, "Blue"=107}, {"Red"=108, "Green"=108, "Blue"=108}, {"Red"=109, "Green"=109, "Blue"=109}, {"Red"=110, "Green"=110, "Blue"=110}, {"Red"=111, "Green"=111, "Blue"=111}, {"Red"=112, "Green"=112, "Blue"=112}, {"Red"=113, "Green"=113, "Blue"=113}, {"Red"=114, "Green"=114, "Blue"=114}, {"Red"=115, "Green"=115, "Blue"=115}, {"Red"=116, "Green"=116, "Blue"=116}, {"Red"=117, "Green"=117, "Blue"=117}, {"Red"=118, "Green"=118, "Blue"=118}, {"Red"=119, "Green"=119, "Blue"=119}, {"Red"=120, "Green"=120, "Blue"=120}, {"Red"=121, "Green"=121, "Blue"=121}, {"Red"=122, "Green"=122, "Blue"=122}, {"Red"=123, "Green"=123, "Blue"=123}, {"Red"=124, "Green"=124, "Blue"=124}, {"Red"=125, "Green"=125, "Blue"=125}, {"Red"=126, "Green"=126, "Blue"=126}, {"Red"=127, "Green"=127, "Blue"=127}, {"Red"=128, "Green"=128, "Blue"=128}, {"Red"=129, "Green"=129, "Blue"=129}, {"Red"=130, "Green"=130, "Blue"=130}, {"Red"=131, "Green"=131, "Blue"=131}, {"Red"=132, "Green"=132, "Blue"=132}, {"Red"=133, "Green"=133, "Blue"=133}, {"Red"=134, "Green"=134, "Blue"=134}, {"Red"=135, "Green"=135, "Blue"=135}, {"Red"=136, "Green"=136, "Blue"=136}, {"Red"=137, "Green"=137, "Blue"=137}, {"Red"=138, "Green"=138, "Blue"=138}, {"Red"=139, "Green"=139, "Blue"=139}, {"Red"=140, "Green"=140, "Blue"=140}, {"Red"=141, "Green"=141, "Blue"=141}, {"Red"=142, "Green"=142, "Blue"=142}, {"Red"=143, "Green"=143, "Blue"=143}, {"Red"=144, "Green"=144, "Blue"=144}, {"Red"=145, "Green"=145, "Blue"=145}, {"Red"=146, "Green"=146, "Blue"=146}, {"Red"=147, "Green"=147, "Blue"=147}, {"Red"=148, "Green"=148, "Blue"=148}, {"Red"=149, "Green"=149, "Blue"=149}, {"Red"=150, "Green"=150, "Blue"=150}, {"Red"=151, "Green"=151, "Blue"=151}, {"Red"=152, "Green"=152, "Blue"=152}, {"Red"=153, "Green"=153, "Blue"=153}, {"Red"=154, "Green"=154, "Blue"=154}, {"Red"=155, "Green"=155, "Blue"=155}, {"Red"=156, "Green"=156, "Blue"=156}, {"Red"=157, "Green"=157, "Blue"=157}, {"Red"=158, "Green"=158, "Blue"=158}, {"Red"=159, "Green"=159, "Blue"=159}, {"Red"=160, "Green"=160, "Blue"=160}, {"Red"=161, "Green"=161, "Blue"=161}, {"Red"=162, "Green"=162, "Blue"=162}, {"Red"=163, "Green"=163, "Blue"=163}, {"Red"=164, "Green"=164, "Blue"=164}, {"Red"=165, "Green"=165, "Blue"=165}, {"Red"=166, "Green"=166, "Blue"=166}, {"Red"=167, "Green"=167, "Blue"=167}, {"Red"=168, "Green"=168, "Blue"=168}, {"Red"=169, "Green"=169, "Blue"=169}, {"Red"=170, "Green"=170, "Blue"=170}, {"Red"=171, "Green"=171, "Blue"=171}, {"Red"=172, "Green"=172, "Blue"=172}, {"Red"=173, "Green"=173, "Blue"=173}, {"Red"=174, "Green"=174, "Blue"=174}, {"Red"=175, "Green"=175, "Blue"=175}, {"Red"=176, "Green"=176, "Blue"=176}, {"Red"=177, "Green"=177, "Blue"=177}, {"Red"=178, "Green"=178, "Blue"=178}, {"Red"=179, "Green"=179, "Blue"=179}, {"Red"=180, "Green"=180, "Blue"=180}, {"Red"=181, "Green"=181, "Blue"=181}, {"Red"=182, "Green"=182, "Blue"=182}, {"Red"=183, "Green"=183, "Blue"=183}, {"Red"=184, "Green"=184, "Blue"=184}, {"Red"=185, "Green"=185, "Blue"=185}, {"Red"=186, "Green"=186, "Blue"=186}, {"Red"=187, "Green"=187, "Blue"=187}, {"Red"=188, "Green"=188, "Blue"=188}, {"Red"=189, "Green"=189, "Blue"=189}, {"Red"=190, "Green"=190, "Blue"=190}, {"Red"=191, "Green"=191, "Blue"=191}, {"Red"=192, "Green"=192, "Blue"=192}, {"Red"=193, "Green"=193, "Blue"=193}, {"Red"=194, "Green"=194, "Blue"=194}, {"Red"=195, "Green"=195, "Blue"=195}, {"Red"=196, "Green"=196, "Blue"=196}, {"Red"=197, "Green"=197, "Blue"=197}, {"Red"=198, "Green"=198, "Blue"=198}, {"Red"=199, "Green"=199, "Blue"=199}, {"Red"=200, "Green"=200, "Blue"=200}, {"Red"=201, "Green"=201, "Blue"=201}, {"Red"=202, "Green"=202, "Blue"=202}, {"Red"=203, "Green"=203, "Blue"=203}, {"Red"=204, "Green"=204, "Blue"=204}, {"Red"=205, "Green"=205, "Blue"=205}, {"Red"=206, "Green"=206, "Blue"=206}, {"Red"=207, "Green"=207, "Blue"=207}, {"Red"=208, "Green"=208, "Blue"=208}, {"Red"=209, "Green"=209, "Blue"=209}, {"Red"=210, "Green"=210, "Blue"=210}, {"Red"=211, "Green"=211, "Blue"=211}, {"Red"=212, "Green"=212, "Blue"=212}, {"Red"=213, "Green"=213, "Blue"=213}, {"Red"=214, "Green"=214, "Blue"=214}, {"Red"=215, "Green"=215, "Blue"=215}, {"Red"=216, "Green"=216, "Blue"=216}, {"Red"=217, "Green"=217, "Blue"=217}, {"Red"=218, "Green"=218, "Blue"=218}, {"Red"=219, "Green"=219, "Blue"=219}, {"Red"=220, "Green"=220, "Blue"=220}, {"Red"=221, "Green"=221, "Blue"=221}, {"Red"=222, "Green"=222, "Blue"=222}, {"Red"=223, "Green"=223, "Blue"=223}, {"Red"=224, "Green"=224, "Blue"=224}, {"Red"=225, "Green"=225, "Blue"=225}, {"Red"=226, "Green"=226, "Blue"=226}, {"Red"=227, "Green"=227, "Blue"=227}, {"Red"=228, "Green"=228, "Blue"=228}, {"Red"=229, "Green"=229, "Blue"=229}, {"Red"=230, "Green"=230, "Blue"=230}, {"Red"=231, "Green"=231, "Blue"=231}, {"Red"=232, "Green"=232, "Blue"=232}, {"Red"=233, "Green"=233, "Blue"=233}, {"Red"=234, "Green"=234, "Blue"=234}, {"Red"=235, "Green"=235, "Blue"=235}, {"Red"=236, "Green"=236, "Blue"=236}, {"Red"=237, "Green"=237, "Blue"=237}, {"Red"=238, "Green"=238, "Blue"=238}, {"Red"=239, "Green"=239, "Blue"=239}, {"Red"=240, "Green"=240, "Blue"=240}, {"Red"=241, "Green"=241, "Blue"=241}, {"Red"=242, "Green"=242, "Blue"=242}, {"Red"=243, "Green"=243, "Blue"=243}, {"Red"=244, "Green"=244, "Blue"=244}, {"Red"=245, "Green"=245, "Blue"=245}, {"Red"=246, "Green"=246, "Blue"=246}, {"Red"=247, "Green"=247, "Blue"=247}, {"Red"=248, "Green"=248, "Blue"=248}, {"Red"=249, "Green"=249, "Blue"=249}, {"Red"=250, "Green"=250, "Blue"=250}, {"Red"=251, "Green"=251, "Blue"=251}, {"Red"=252, "Green"=252, "Blue"=252}, {"Red"=253, "Green"=253, "Blue"=253}, {"Red"=254, "Green"=254, "Blue"=254}, {"Red"=255, "Green"=0, "Blue"=0}] ("Color Palette") cluster{"Red":u8, "Green":u8, "Blue":u8}[] [{"Red"=0, "Green"=0, "Blue"=0}, {"Red"=1, "Green"=1, "Blue"=1}, {"Red"=2, "Green"=2, "Blue"=2}, {"Red"=3, "Green"=3, "Blue"=3}, {"Red"=4, "Green"=4, "Blue"=4}, {"Red"=5, "Green"=5, "Blue"=5}, {"Red"=6, "Green"=6, "Blue"=6}, {"Red"=7, "Green"=7, "Blue"=7}, {"Red"=8, "Green"=8, "Blue"=8}, {"Red"=9, "Green"=9, "Blue"=9}, {"Red"=10, "Green"=10, "Blue"=10}, {"Red"=11, "Green"=11, "Blue"=11}, {"Red"=12, "Green"=12, "Blue"=12}, {"Red"=13, "Green"=13, "Blue"=13}, {"Red"=14, "Green"=14, "Blue"=14}, {"Red"=15, "Green"=15, "Blue"=15}, {"Red"=16, "Green"=16, "Blue"=16}, {"Red"=17, "Green"=17, "Blue"=17}, {"Red"=18, "Green"=18, "Blue"=18}, {"Red"=19, "Green"=19, "Blue"=19}, {"Red"=20, "Green"=20, "Blue"=20}, {"Red"=21, "Green"=21, "Blue"=21}, {"Red"=22, "Green"=22, "Blue"=22}, {"Red"=23, "Green"=23, "Blue"=23}, {"Red"=24, "Green"=24, "Blue"=24}, {"Red"=25, "Green"=25, "Blue"=25}, {"Red"=26, "Green"=26, "Blue"=26}, {"Red"=27, "Green"=27, "Blue"=27}, {"Red"=28, "Green"=28, "Blue"=28}, {"Red"=29, "Green"=29, "Blue"=29}, {"Red"=30, "Green"=30, "Blue"=30}, {"Red"=31, "Green"=31, "Blue"=31}, {"Red"=32, "Green"=32, "Blue"=32}, {"Red"=33, "Green"=33, "Blue"=33}, {"Red"=34, "Green"=34, "Blue"=34}, {"Red"=35, "Green"=35, "Blue"=35}, {"Red"=36, "Green"=36, "Blue"=36}, {"Red"=37, "Green"=37, "Blue"=37}, {"Red"=38, "Green"=38, "Blue"=38}, {"Red"=39, "Green"=39, "Blue"=39}, {"Red"=40, "Green"=40, "Blue"=40}, {"Red"=41, "Green"=41, "Blue"=41}, {"Red"=42, "Green"=42, "Blue"=42}, {"Red"=43, "Green"=43, "Blue"=43}, {"Red"=44, "Green"=44, "Blue"=44}, {"Red"=45, "Green"=45, "Blue"=45}, {"Red"=46, "Green"=46, "Blue"=46}, {"Red"=47, "Green"=47, "Blue"=47}, {"Red"=48, "Green"=48, "Blue"=48}, {"Red"=49, "Green"=49, "Blue"=49}, {"Red"=50, "Green"=50, "Blue"=50}, {"Red"=51, "Green"=51, "Blue"=51}, {"Red"=52, "Green"=52, "Blue"=52}, {"Red"=53, "Green"=53, "Blue"=53}, {"Red"=54, "Green"=54, "Blue"=54}, {"Red"=55, "Green"=55, "Blue"=55}, {"Red"=56, "Green"=56, "Blue"=56}, {"Red"=57, "Green"=57, "Blue"=57}, {"Red"=58, "Green"=58, "Blue"=58}, {"Red"=59, "Green"=59, "Blue"=59}, {"Red"=60, "Green"=60, "Blue"=60}, {"Red"=61, "Green"=61, "Blue"=61}, {"Red"=62, "Green"=62, "Blue"=62}, {"Red"=63, "Green"=63, "Blue"=63}, {"Red"=64, "Green"=64, "Blue"=64}, {"Red"=65, "Green"=65, "Blue"=65}, {"Red"=66, "Green"=66, "Blue"=66}, {"Red"=67, "Green"=67, "Blue"=67}, {"Red"=68, "Green"=68, "Blue"=68}, {"Red"=69, "Green"=69, "Blue"=69}, {"Red"=70, "Green"=70, "Blue"=70}, {"Red"=71, "Green"=71, "Blue"=71}, {"Red"=72, "Green"=72, "Blue"=72}, {"Red"=73, "Green"=73, "Blue"=73}, {"Red"=74, "Green"=74, "Blue"=74}, {"Red"=75, "Green"=75, "Blue"=75}, {"Red"=76, "Green"=76, "Blue"=76}, {"Red"=77, "Green"=77, "Blue"=77}, {"Red"=78, "Green"=78, "Blue"=78}, {"Red"=79, "Green"=79, "Blue"=79}, {"Red"=80, "Green"=80, "Blue"=80}, {"Red"=81, "Green"=81, "Blue"=81}, {"Red"=82, "Green"=82, "Blue"=82}, {"Red"=83, "Green"=83, "Blue"=83}, {"Red"=84, "Green"=84, "Blue"=84}, {"Red"=85, "Green"=85, "Blue"=85}, {"Red"=86, "Green"=86, "Blue"=86}, {"Red"=87, "Green"=87, "Blue"=87}, {"Red"=88, "Green"=88, "Blue"=88}, {"Red"=89, "Green"=89, "Blue"=89}, {"Red"=90, "Green"=90, "Blue"=90}, {"Red"=91, "Green"=91, "Blue"=91}, {"Red"=92, "Green"=92, "Blue"=92}, {"Red"=93, "Green"=93, "Blue"=93}, {"Red"=94, "Green"=94, "Blue"=94}, {"Red"=95, "Green"=95, "Blue"=95}, {"Red"=96, "Green"=96, "Blue"=96}, {"Red"=97, "Green"=97, "Blue"=97}, {"Red"=98, "Green"=98, "Blue"=98}, {"Red"=99, "Green"=99, "Blue"=99}, {"Red"=100, "Green"=100, "Blue"=100}, {"Red"=101, "Green"=101, "Blue"=101}, {"Red"=102, "Green"=102, "Blue"=102}, {"Red"=103, "Green"=103, "Blue"=103}, {"Red"=104, "Green"=104, "Blue"=104}, {"Red"=105, "Green"=105, "Blue"=105}, {"Red"=106, "Green"=106, "Blue"=106}, {"Red"=107, "Green"=107, "Blue"=107}, {"Red"=108, "Green"=108, "Blue"=108}, {"Red"=109, "Green"=109, "Blue"=109}, {"Red"=110, "Green"=110, "Blue"=110}, {"Red"=111, "Green"=111, "Blue"=111}, {"Red"=112, "Green"=112, "Blue"=112}, {"Red"=113, "Green"=113, "Blue"=113}, {"Red"=114, "Green"=114, "Blue"=114}, {"Red"=115, "Green"=115, "Blue"=115}, {"Red"=116, "Green"=116, "Blue"=116}, {"Red"=117, "Green"=117, "Blue"=117}, {"Red"=118, "Green"=118, "Blue"=118}, {"Red"=119, "Green"=119, "Blue"=119}, {"Red"=120, "Green"=120, "Blue"=120}, {"Red"=121, "Green"=121, "Blue"=121}, {"Red"=122, "Green"=122, "Blue"=122}, {"Red"=123, "Green"=123, "Blue"=123}, {"Red"=124, "Green"=124, "Blue"=124}, {"Red"=125, "Green"=125, "Blue"=125}, {"Red"=126, "Green"=126, "Blue"=126}, {"Red"=127, "Green"=127, "Blue"=127}, {"Red"=128, "Green"=128, "Blue"=128}, {"Red"=129, "Green"=129, "Blue"=129}, {"Red"=130, "Green"=130, "Blue"=130}, {"Red"=131, "Green"=131, "Blue"=131}, {"Red"=132, "Green"=132, "Blue"=132}, {"Red"=133, "Green"=133, "Blue"=133}, {"Red"=134, "Green"=134, "Blue"=134}, {"Red"=135, "Green"=135, "Blue"=135}, {"Red"=136, "Green"=136, "Blue"=136}, {"Red"=137, "Green"=137, "Blue"=137}, {"Red"=138, "Green"=138, "Blue"=138}, {"Red"=139, "Green"=139, "Blue"=139}, {"Red"=140, "Green"=140, "Blue"=140}, {"Red"=141, "Green"=141, "Blue"=141}, {"Red"=142, "Green"=142, "Blue"=142}, {"Red"=143, "Green"=143, "Blue"=143}, {"Red"=144, "Green"=144, "Blue"=144}, {"Red"=145, "Green"=145, "Blue"=145}, {"Red"=146, "Green"=146, "Blue"=146}, {"Red"=147, "Green"=147, "Blue"=147}, {"Red"=148, "Green"=148, "Blue"=148}, {"Red"=149, "Green"=149, "Blue"=149}, {"Red"=150, "Green"=150, "Blue"=150}, {"Red"=151, "Green"=151, "Blue"=151}, {"Red"=152, "Green"=152, "Blue"=152}, {"Red"=153, "Green"=153, "Blue"=153}, {"Red"=154, "Green"=154, "Blue"=154}, {"Red"=155, "Green"=155, "Blue"=155}, {"Red"=156, "Green"=156, "Blue"=156}, {"Red"=157, "Green"=157, "Blue"=157}, {"Red"=158, "Green"=158, "Blue"=158}, {"Red"=159, "Green"=159, "Blue"=159}, {"Red"=160, "Green"=160, "Blue"=160}, {"Red"=161, "Green"=161, "Blue"=161}, {"Red"=162, "Green"=162, "Blue"=162}, {"Red"=163, "Green"=163, "Blue"=163}, {"Red"=164, "Green"=164, "Blue"=164}, {"Red"=165, "Green"=165, "Blue"=165}, {"Red"=166, "Green"=166, "Blue"=166}, {"Red"=167, "Green"=167, "Blue"=167}, {"Red"=168, "Green"=168, "Blue"=168}, {"Red"=169, "Green"=169, "Blue"=169}, {"Red"=170, "Green"=170, "Blue"=170}, {"Red"=171, "Green"=171, "Blue"=171}, {"Red"=172, "Green"=172, "Blue"=172}, {"Red"=173, "Green"=173, "Blue"=173}, {"Red"=174, "Green"=174, "Blue"=174}, {"Red"=175, "Green"=175, "Blue"=175}, {"Red"=176, "Green"=176, "Blue"=176}, {"Red"=177, "Green"=177, "Blue"=177}, {"Red"=178, "Green"=178, "Blue"=178}, {"Red"=179, "Green"=179, "Blue"=179}, {"Red"=180, "Green"=180, "Blue"=180}, {"Red"=181, "Green"=181, "Blue"=181}, {"Red"=182, "Green"=182, "Blue"=182}, {"Red"=183, "Green"=183, "Blue"=183}, {"Red"=184, "Green"=184, "Blue"=184}, {"Red"=185, "Green"=185, "Blue"=185}, {"Red"=186, "Green"=186, "Blue"=186}, {"Red"=187, "Green"=187, "Blue"=187}, {"Red"=188, "Green"=188, "Blue"=188}, {"Red"=189, "Green"=189, "Blue"=189}, {"Red"=190, "Green"=190, "Blue"=190}, {"Red"=191, "Green"=191, "Blue"=191}, {"Red"=192, "Green"=192, "Blue"=192}, {"Red"=193, "Green"=193, "Blue"=193}, {"Red"=194, "Green"=194, "Blue"=194}, {"Red"=195, "Green"=195, "Blue"=195}, {"Red"=196, "Green"=196, "Blue"=196}, {"Red"=197, "Green"=197, "Blue"=197}, {"Red"=198, "Green"=198, "Blue"=198}, {"Red"=199, "Green"=199, "Blue"=199}, {"Red"=200, "Green"=200, "Blue"=200}, {"Red"=201, "Green"=201, "Blue"=201}, {"Red"=202, "Green"=202, "Blue"=202}, {"Red"=203, "Green"=203, "Blue"=203}, {"Red"=204, "Green"=204, "Blue"=204}, {"Red"=205, "Green"=205, "Blue"=205}, {"Red"=206, "Green"=206, "Blue"=206}, {"Red"=207, "Green"=207, "Blue"=207}, {"Red"=208, "Green"=208, "Blue"=208}, {"Red"=209, "Green"=209, "Blue"=209}, {"Red"=210, "Green"=210, "Blue"=210}, {"Red"=211, "Green"=211, "Blue"=211}, {"Red"=212, "Green"=212, "Blue"=212}, {"Red"=213, "Green"=213, "Blue"=213}, {"Red"=214, "Green"=214, "Blue"=214}, {"Red"=215, "Green"=215, "Blue"=215}, {"Red"=216, "Green"=216, "Blue"=216}, {"Red"=217, "Green"=217, "Blue"=217}, {"Red"=218, "Green"=218, "Blue"=218}, {"Red"=219, "Green"=219, "Blue"=219}, {"Red"=220, "Green"=220, "Blue"=220}, {"Red"=221, "Green"=221, "Blue"=221}, {"Red"=222, "Green"=222, "Blue"=222}, {"Red"=223, "Green"=223, "Blue"=223}, {"Red"=224, "Green"=224, "Blue"=224}, {"Red"=225, "Green"=225, "Blue"=225}, {"Red"=226, "Green"=226, "Blue"=226}, {"Red"=227, "Green"=227, "Blue"=227}, {"Red"=228, "Green"=228, "Blue"=228}, {"Red"=229, "Green"=229, "Blue"=229}, {"Red"=230, "Green"=230, "Blue"=230}, {"Red"=231, "Green"=231, "Blue"=231}, {"Red"=232, "Green"=232, "Blue"=232}, {"Red"=233, "Green"=233, "Blue"=233}, {"Red"=234, "Green"=234, "Blue"=234}, {"Red"=235, "Green"=235, "Blue"=235}, {"Red"=236, "Green"=236, "Blue"=236}, {"Red"=237, "Green"=237, "Blue"=237}, {"Red"=238, "Green"=238, "Blue"=238}, {"Red"=239, "Green"=239, "Blue"=239}, {"Red"=240, "Green"=240, "Blue"=240}, {"Red"=241, "Green"=241, "Blue"=241}, {"Red"=242, "Green"=242, "Blue"=242}, {"Red"=243, "Green"=243, "Blue"=243}, {"Red"=244, "Green"=244, "Blue"=244}, {"Red"=245, "Green"=245, "Blue"=245}, {"Red"=246, "Green"=246, "Blue"=246}, {"Red"=247, "Green"=247, "Blue"=247}, {"Red"=248, "Green"=248, "Blue"=248}, {"Red"=249, "Green"=249, "Blue"=249}, {"Red"=250, "Green"=250, "Blue"=250}, {"Red"=251, "Green"=251, "Blue"=251}, {"Red"=252, "Green"=252, "Blue"=252}, {"Red"=253, "Green"=253, "Blue"=253}, {"Red"=254, "Green"=254, "Blue"=254}, {"Red"=255, "Green"=255, "Blue"=255}] ("Color Palette")] -> w93
              frame "high clipping red" {
              }
              frame "low clipping blue" {
              }
              frame "high and low clipping" {
              }
              frame "standard" {
              }
            }
            n54 = call-poly "GFGpolyGet.vi"() -> ("error out"=w98:errorcluster, "DisplayRefsOut(generic class)"=w97:T13)  [unwired: 10 in]
            n55 = Cluster To Array(cluster=w97) -> (array=w95:refnum<vi>[])
            n56 = for {
              tunnel: w95 -> [w108] mode=indexing
              tunnel: w93 -> [w104]
              tunnel: w94 -> [w103]
              tunnel: w98 -> [w105]
              tunnel: w96 -> [w107]
              n57 = To More Specific Class(target class=w107, reference=w108) -> (specific class reference=w106:refnum<vi>)  [unwired: 1 in, 1 out]
              n58 = property class="ImageControl"(reference=w106, error in=w105, "User Palette"=w104, "Palette Type"=w103) -> ()  [unwired: 2 out]
            }
          }
          frame "no..of.frames.to.acquire" {
            n59 = Variant To Data(type=0.0, Variant=w121) -> (data=w115:dbl)  [unwired: 1 in, 1 out]
            n60 = call-poly "GFGpolyGet.vi"("Variable Name in"="frame count") -> ("output cluster"=w123:T12)  [unwired: 9 in, 1 out]
            n61 = call "GFG_core.vi"("Variable Name in"="scan mode main settings") -> ("Variant Out"=w117:variant)  [unwired: 12 in, 6 out]
            n62 = Unbundle By Name(w123) -> ("SlideRef"=w122:refnum<vi>)
            n63 = Variant To Data(type=scan_mode_main_settings_tab."2D line scan" ("scan mode main settings"), Variant=w117) -> (data=w114:T2)  [unwired: 1 in, 1 out]
            n64 = property class="Slide"(reference=w122, "Scale.Maximum"=w115) -> ()  [unwired: 1 in, 2 out]
            n65 = case shown="\"2D frame\", Default" w114 {
              tunnel: w115 -> [w125 _]
              frame "2D frame", Default {
                n66 = call "GFG_core.vi"("Variable Name in"="no.of.frames.for.frame.scan", "Variant in"=w125, "Action"=enum16{"Init", "Set", "Get"}."Set") -> ()  [unwired: 10 in, 7 out]
              }
              frame "2D line scan" {
              }
            }
          }
          frame "piezo.mode" {
            n67 = call-poly "GFGpolyGet.vi"("Variable Name in"="frames.per.z.cycle") -> ("output cluster"=w136:T12)  [unwired: 9 in, 1 out]
            n68 = call-poly "GFGpolyGet.vi"("Variable Name in"="piezo.mode") -> ("Boolean"=w130:bool)  [unwired: 10 in]
            n69 = Unbundle By Name(w136) -> ("DigitalRef"=w135:refnum<vi>)
            n70 = Select(t=T4 {"Minimum"=3.0, "Maximum"=101.0, "Increment"=2.0} ("Data Entry Limits"), s=w130, f=T4 {"Minimum"=4.0, "Maximum"=100.0, "Increment"=2.0} ("Data Entry Limits")) -> (s? t:f=w131:T4)
            n71 = property class="DigNum"(reference=w135, "Data Range"=w131, "OutOfRngAction"=T3 {"Out of Range Action Minimum"=1, "Out of Range Action Maximum"=1, "Out of Range Action Increment"=1} ("Response to Value Outside Limits")) -> ()  [unwired: 1 in, 2 out]
          }
          frame "Start.Delay", "ZOOM", "pixel.resolution", "speed.mode" {
            n72 = flat-sequence {
              tunnel: w142 -> [w150]
              tunnel: w141 -> [w148]
              tunnel: [w147] -> w140
              tunnel: w140 -> [w152]
              tunnel: [w151] -> w139
              frame #0 {
                n73 = Wait (ms)(milliseconds to wait=u32 30) -> ()  [unwired: 1 out]
              }
              frame #1 {
                n74 = call "GFG_core.vi"("Variable Name in"=w150) -> ("Variant Out"=w149:variant)  [unwired: 12 in, 6 out]
                n75 = Equal?(x=w149, y=w148) -> (x = y?=w147:bool)
              }
              frame #2 {
                n76 = case shown="True" w152 {
                  tunnel: [_ w154] -> w151
                  frame False {
                  }
                  frame True {
                    n77 = call-poly "GFGpolyGet.vi"("Variable Name in"="FOCUS") -> ("Boolean"=w153:bool)  [unwired: 10 in]
                    n78 = case shown="True" w153 {
                      frame False {
                      }
                      frame True {
                        n79 = Build Array("Start.Delay" ("Variable Name in"), "ZOOM" ("Variable Name in"), "x.correction" ("Variable Name in")) -> (w162:string[])
                        n80 = for {
                          tunnel: w162 -> [w163] mode=indexing
                          n81 = call-poly "GFGpolyGet.vi"("Variable Name in"=w163) -> ("output cluster"=w166:T12)  [unwired: 9 in, 1 out]
                          n82 = Unbundle By Name(w166) -> ("SlideRef"=w164:refnum<vi>)
                          n83 = property class="Slide"(reference=w164, "DisabledEnum"=T5."Disabled" ("Disabled")) -> ()  [unwired: 1 in, 2 out]
                        }
                      }
                    }
                    n84 = call "GFG_core.vi"("Variable Name in"="flystop", "Variant in"=w153, "Action"=enum16{"Init", "Set", "Get"}."Set") -> ("error out"=w154:errorcluster)  [unwired: 10 in, 6 out]
                    n85 = Wait (ms)(milliseconds to wait=u32 50) -> ()  [unwired: 1 out]
                  }
                }
              }
            }
            n86 = case shown="\"pixel.resolution\"" w142 {
              tunnel: w141 -> [_ _ _ w273]
              tunnel: [w243 w251 w264 w271] -> w145
              tunnel: w139 -> [_ _ _ _]
              frame "ZOOM", Default {
                n87 = call "GFG_core.vi"("Variable Name in"="pixel.resolution") -> ("Variant Out"=w245:variant)  [unwired: 12 in, 6 out]
                n88 = Variant To Data(type=pixel_resolution_enum."   128 x 128" ("pixel resolution"), Variant=w245) -> (data=w243:T6)  [unwired: 1 in, 1 out]
              }
              frame "x.correction" {
                n89 = call-poly "GFGpolyGet.vi"("Variable Name in"="x.correction") -> ("Numeric"=w247:dbl)  [unwired: 9 in, 1 out]
                n90 = call-poly "GFGpolyGet.vi"("Variable Name in"="resonant.correction.enable") -> ("Boolean"=w250:bool)  [unwired: 10 in]
                n91 = case shown="False" w250 {
                  tunnel: ["x.correction.shift" ("Variable Name in") "x.correction.cosine" ("Variable Name in")] -> w248
                  frame False {
                  }
                  frame True {
                  }
                }
                n92 = call "GFG_core.vi"("Variable Name in"=w248, "Variant in"=w247, "Action"=enum16{"Init", "Set", "Get"}."Set") -> ()  [unwired: 10 in, 7 out]
                n93 = call "GFG_core.vi"("Variable Name in"="pixel.resolution") -> ("Variant Out"=w253:variant)  [unwired: 12 in, 6 out]
                n94 = Variant To Data(type=pixel_resolution_enum."   128 x 128" ("pixel resolution"), Variant=w253) -> (data=w251:T6)  [unwired: 1 in, 1 out]
              }
              frame "resonant.correction.enable" {
                n95 = call-poly "GFGpolyGet.vi"("Variable Name in"="resonant.correction.enable") -> ("Boolean"=w263:bool)  [unwired: 10 in]
                n96 = case shown="False" w263 {
                  tunnel: ["x.correction.shift" ("Variable Name in") "x.correction.cosine" ("Variable Name in")] -> w260
                  frame False {
                  }
                  frame True {
                  }
                }
                n97 = call-poly "GFGpolyGet.vi"("Variable Name in"=w260) -> ("Numeric"=w261:dbl)  [unwired: 9 in, 1 out]
                n98 = call "GFG_core.vi"("Variable Name in"="x.correction", "Variant in"=w261, "Action"=enum16{"Init", "Set", "Get"}."Set") -> ()  [unwired: 10 in, 7 out]
                n99 = call "GFG_core.vi"("Variable Name in"="pixel.resolution") -> ("Variant Out"=w266:variant)  [unwired: 12 in, 6 out]
                n100 = Variant To Data(type=pixel_resolution_enum."   128 x 128" ("pixel resolution"), Variant=w266) -> (data=w264:T6)  [unwired: 1 in, 1 out]
              }
              frame "pixel.resolution" {
                n101 = Variant To Data(type=pixel_resolution_enum."   128 x 128" ("pixel resolution"), Variant=w273) -> (data=w271:T6)  [unwired: 1 in, 1 out]
              }
            }
            n102 = case shown="Default" w145 {
              selector: w145 -> [_ w216]
              frame "   arbitrary" {
                w169 = "nomin.x.pixels" ("Variable Name in")
                n103 = call-poly "GFGpolyGet.vi"("Variable Name in"="ZOOM") -> ("output cluster"=w174:T12)  [unwired: 9 in, 1 out]
                n104 = call-poly "GFGpolyGet.vi"("Variable Name in"="speed.mode") -> ("output cluster"=w179:T12)  [unwired: 9 in, 1 out]
                n105 = Build Array("nomin.x.pixels" ("Variable Name in"), "y.pixel.sz" ("Variable Name in"), "x.pixel.sz" ("Variable Name in"), "pixel.dwell.time.in.sec" ("Variable Name in")) -> (w180:string[])
                n106 = Unbundle By Name(w174) -> ("SlideRef"=w176:refnum<vi>)
                n107 = Unbundle By Name(w179) -> ("RingRef"=w177:refnum<vi>)
                n108 = property class="Slide"(reference=w176, "DisabledEnum"=T5."Disabled and Grayed Out" ("Disabled")) -> ()  [unwired: 1 in, 2 out]
                n109 = property class="Ring"(reference=w177, "DisabledEnum"=T5."Disabled and Grayed Out" ("Disabled")) -> ()  [unwired: 1 in, 2 out]
                n110 = for {
                  tunnel: w180 -> [w187] mode=indexing
                  n111 = call-poly "GFGpolyGet.vi"("Variable Name in"=w187) -> ("output cluster"=w186:T12)  [unwired: 9 in, 1 out]
                  n112 = Unbundle By Name(w186) -> ("DigitalRef"=w184:refnum<vi>)
                  n113 = property class="DigNum"(reference=w184, "DisabledEnum"=T5."Enabled" ("Disabled")) -> ()  [unwired: 1 in, 2 out]
                }
                n114 = call "GFG_core.vi"("Variable Name in"=w169, "Action"=enum16{"Init", "Set", "Get"}."Get") -> ("Variant Out"=w168:variant)  [unwired: 11 in, 6 out]
                n115 = call "GFG_core.vi"("Variable Name in"=w169, "Variant in"=w168, "Action"=enum16{"Init", "Set", "Get"}."Set") -> ()  [unwired: 10 in, 7 out]
              }
              frame Default {
                n116 = Build Array("nomin.x.pixels" ("Variable Name in"), "y.pixel.sz" ("Variable Name in"), "x.pixel.sz" ("Variable Name in")) -> (w210:string[])
                n117 = for {
                  tunnel: w210 -> [w242] mode=indexing
                  n118 = call-poly "GFGpolyGet.vi"("Variable Name in"=w242) -> ("output cluster"=w241:T12)  [unwired: 9 in, 1 out]
                  n119 = Unbundle By Name(w241) -> ("DigitalRef"=w239:refnum<vi>)
                  n120 = property class="DigNum"(reference=w239, "DisabledEnum"=T5."Disabled and Grayed Out" ("Disabled")) -> ()  [unwired: 1 in, 2 out]
                }
                n121 = case shown="\"   512 x 512\"" w216 {
                  tunnel: [128 256 256 512 512 512 512 1024 1024] -> w188
                  tunnel: [128 128 256 256 128 64 512 512 1024] -> w191
                  frame "   128 x 128", Default {
                  }
                  frame "   256 x 128" {
                  }
                  frame "   256 x 256" {
                  }
                  frame "   512 x 256" {
                  }
                  frame "   512 x 128" {
                  }
                  frame "   512 x  64" {
                  }
                  frame "   512 x 512" {
                  }
                  frame "  1024 x 512" {
                  }
                  frame "  1024 x 1024" {
                  }
                }
                n122 = call "GFG_core.vi"("Variable Name in"="y.pixels", "Variant in"=w191, "Action"=enum16{"Init", "Set", "Get"}."Set") -> ()  [unwired: 10 in, 7 out]
                n123 = disable-structure shown="Disabled" {
                  frame Disabled {
                    n124 = call-poly "GFGpolyGet.vi"("Variable Name in"="ZOOM") -> ("output cluster"=w218:T12)  [unwired: 9 in, 1 out]
                    n125 = Unbundle By Name(w218) -> ("SlideRef"=w220:refnum<vi>)
                    n126 = property class="Slide"(reference=w220, "DisabledEnum"=T5."Enabled" ("Disabled")) -> ()  [unwired: 1 in, 2 out]
                  }
                  frame Enabled {
                  }
                }
                n127 = call-poly "GFGpolyGet.vi"("Variable Name in"="max.field.of.view.resonant") -> ("Numeric"=w195:dbl)  [unwired: 9 in, 1 out]
                n128 = call-poly "GFGpolyGet.vi"("Variable Name in"="max.field.of.view") -> ("Numeric"=w207:dbl)  [unwired: 9 in, 1 out]
                n129 = Build Array(w188, w191) -> (w199:i32[])
                n130 = call-poly "GFGpolyGet.vi"("Variable Name in"="ZOOM") -> ("Numeric"=w196:dbl)  [unwired: 9 in, 1 out]
                n131 = Divide(x=w207, y=w196) -> (x/y=w200:dbl)
                n132 = Divide(x=w195, y=w196) -> (x/y=w194:dbl)
                n133 = Array Max & Min(array=w199) -> (max value=w192:i32)  [unwired: 3 out]
                n134 = Divide(x=w194, y=w188) -> (x/y=w193:dbl)
                n135 = Divide(x=w200, y=w192) -> (x/y=w198:dbl)
                n136 = call "GFG_core.vi"("Variable Name in"="x.pixel.sz", "Variant in"=w193, "Action"=enum16{"Init", "Set", "Get"}."Set") -> ()  [unwired: 10 in, 7 out]
                n137 = call "GFG_core.vi"("Variable Name in"="x.pixels", "Variant in"=w188, "Action"=enum16{"Init", "Set", "Get"}."Set") -> ()  [unwired: 10 in, 7 out]
                n138 = call "GFG_core.vi"("Variable Name in"="y.pixel.sz", "Variant in"=w198, "Action"=enum16{"Init", "Set", "Get"}."Set") -> ()  [unwired: 10 in, 7 out]
                n139 = call "GFG_core.vi"("Variable Name in"="nomin.x.pixels", "Variant in"=w188, "Action"=enum16{"Init", "Set", "Get"}."Set") -> ()  [unwired: 10 in, 7 out]
              }
            }
          }
          frame "reset.zoom" {
            n140 = call-poly "GFGpolyGet.vi"() -> ("DisplayRefsOut(generic class)"=w280:T13)  [unwired: 10 in, 1 out]
            n141 = call-poly "GFGpolyGet.vi"() -> ("Image Refs Out"=w279:T15)  [unwired: 10 in, 1 out]
            n142 = Cluster To Array(cluster=w280) -> (array=w278:refnum<vi>[])
            n143 = Cluster To Array(cluster=w279) -> (array=w277:T14[])
            n144 = call "set initial zoom.vi"("reset?"=TRUE, "Image Refs In"=w277, "DisplayRefsIn(generic class)"=w278) -> ()  [unwired: 9 in]
          }
          frame "max.field.of.view", "max.field.of.view.resonant", "nomin.x.pixels", "voltage.for.max.field.of.view", "voltage.for.max.field.of.view.resonant", "x.pixel.sz", "x.volt.offset", "y.pixel.sz", "y.pixels", "y.volt.offset" {
            n145 = for {
              N: 1 -> [_]
              shift-right: [w286] -> _
              shift-left: _ -> [w288]
              tunnel: [w285] -> w281
              n146 = Tick Count (ms)() -> (millisecond timer value=w286:u32)
              n147 = Subtract(x=w286, y=w288) -> (x-y=w289:u32)
              n148 = Greater?(x=w289, y=u32 500) -> (0:w285:bool)
            }
            n149 = case shown="True" w281 {
              frame False {
              }
              frame True {
                n150 = call "GFG refresh all variables.vi"("All Variable Names"=string[] ["ZOOM"]) -> ()  [unwired: 11 in]
              }
            }
          }
          frame "scan.mode.main.settings" {
            n151 = Variant To Data(type=scan_mode_main_settings_tab."2D frame" ("scan mode main settings"), Variant=w296) -> (data=w294:T2)  [unwired: 1 in, 1 out]
            n152 = case shown="\"Z Stack\"" w294 {
              tunnel: w293 -> [w311 w322 w329]
              tunnel: [w311 w322 w329] -> w292
              frame "2D frame", Default {
                n153 = call "GFG refresh all variables.vi"("All Variable Names"=string[] ["pixel resolution", "x.bidirectional"]) -> ()  [unwired: 11 in]
                n154 = call "GFG_core.vi"("Variable Name in"="no..of.frames.for.frame.scan", "Action"=enum16{"Init", "Set", "Get"}."Get") -> ("Variable Name Out"=w305:string)  [unwired: 11 in, 6 out]
                n155 = call "GFG_core.vi"("Variable Name in"="experiment type", "Variant in"=T7 "XYT" ("experiment type"), "Action"=enum16{"Init", "Set", "Get"}."Set") -> ()  [unwired: 10 in, 7 out]
                n156 = disable-structure shown="Disabled" {
                  frame Disabled {
                    n157 = call-poly "GFGpolyGet.vi"("Variable Name in"="fill.fraction") -> ("output cluster"=w314:T12)  [unwired: 9 in, 1 out]
                    n158 = Unbundle By Name(w314) -> ("DigitalRef"=w315:refnum<vi>)
                    n159 = property class="DigNum"(reference=w315, "DisabledEnum"=T5."Enabled" ("Disabled")) -> ()  [unwired: 1 in, 2 out]
                  }
                  frame Enabled {
                  }
                }
                n160 = call "GFG_core.vi"("Variable Name in"=" no..of.frames.to.acquire", "Variant in"=w305, "Action"=enum16{"Init", "Set", "Get"}."Set") -> ()  [unwired: 10 in, 7 out]
                n161 = call-poly "GFGpolyGet.vi"("Variable Name in"="y.pixels") -> ("output cluster"=w302:T12)  [unwired: 9 in, 1 out]
                n162 = call "line scan enable disable.vi"("Page Enabled State"=T8."Page Disabled & Grayed") -> ()  [unwired: 11 in]
                n163 = Unbundle By Name(w302) -> ("DigitalRef"=w301:refnum<vi>)
                n164 = property class="DigNum"(reference=w301, "DisabledEnum"=T5."Enabled" ("Disabled")) -> ()  [unwired: 1 in, 2 out]
              }
              frame "Z Stack" {
                n165 = call "GFG_core.vi"("Variable Name in"="experiment type", "Variant in"=T7 "XYTZ" ("experiment type"), "Action"=enum16{"Init", "Set", "Get"}."Set") -> ()  [unwired: 10 in, 7 out]
                n166 = call "GFG_core.vi"("Variable Name in"="advanced settings inner tab", "Variant in"=advanced_settings_inner_tab_CTL."Zstack data" ("advanced settings inner tab"), "Action"=enum16{"Init", "Set", "Get"}."Set") -> ()  [unwired: 10 in, 7 out]
                n167 = call "control tab sliding.vi"("close(T)/open(F)"=FALSE, "String"="advanced settings slider tab") -> ()  [unwired: 10 in]
                n168 = call "GFG refresh all variables.vi"("All Variable Names"=string[] ["frames.per.plane"]) -> ()  [unwired: 11 in]
              }
              frame "2D line scan" {
                n169 = call "GFG_core.vi"("Variable Name in"="experiment type", "Variant in"=T7 "[xy]T" ("experiment type"), "Action"=enum16{"Init", "Set", "Get"}."Set") -> ()  [unwired: 10 in, 7 out]
              }
            }
          }
          frame "resonant.display.queue.to.fp.display_MD.completed", "resonant.image.queue.to.disk.and.display.queue_MD.completed", "resonant.raw.queue.to.image.queue_MD.completed", "resonant.scan.engine_MD.completed" {
            n170 = for {
              N: 1 -> [_]
              shift-right: [w345] -> _
              shift-left: _ -> [w347]
              tunnel: [w346] -> w336
              n171 = Tick Count (ms)() -> (millisecond timer value=w345:u32)
              n172 = Subtract(x=w345, y=w347) -> (x-y=w346:u32)
            }
            n173 = Greater?(x=u32 1000 ("y"), y=w336) -> (0:w333:bool)
            n174 = local read "String"() -> (w332:string)
            n175 = Select(t=w332, s=w333, f="") -> (s? t:f=w334:string)
            n176 = Concatenate Strings(w334, "\r\n", w342) -> (w341:string)
            n177 = for {
              tunnel: w341 -> [w354]
              tunnel: string[] ["resonant.scan.engine_MD.completed", "resonant.raw.queue.to.image.queue_MD.completed", "resonant.image.queue.to.disk.and.display.queue_MD.completed", "resonant.display.queue.to.fp.display_MD.completed"] ("appended array") -> [w353] mode=indexing
              shift-right: [w349] -> w338
              shift-left: i16 0 -> [w348]
              n178 = Match Pattern(string=w354, regular expression=w353) -> (offset past match=w352:i32)  [unwired: 1 in, 3 out]
              n179 = Greater Or Equal To 0?(x=w352) -> (x >= 0?=w351:bool)
              n180 = Boolean To (0,1)(Boolean=w351) -> (0, 1=w350:i16)
              n181 = Add(x=w350, y=w348) -> (x+y=w349:i16)
            }
            n182 = local write "String"(w341) -> ()
            n183 = disable-structure shown="Enabled" {
              disable-tunnel: w338 -> [w356 _]
              frame Enabled {
                n184 = Equal?(x=w356, y=4) -> (x = y?=w355:bool)
                n185 = case shown="True" w355 {
                  selector: w355 -> [_ w358]
                  frame False {
                  }
                  frame True {
                    n186 = local write "String"("") -> ()
                    "ready for flystart?" <- w358
                  }
                }
              }
              frame Disabled {
              }
            }
          }
          frame "MAIN.Image.panels.reso." {
            n187 = Variant To Data(type=MAIN_Image_panel_reso_tab_Control_type_def."Channel 2" ("MAIN Image panels reso"), Variant=w369) -> (data=w368:T10)  [unwired: 1 in, 1 out]
            n188 = case shown="\"Channel 3\"" w368 {
              tunnel: w367 -> [w371 w373 w375 w377 w379]
              tunnel: [w371 w373 w375 w377 w379] -> w366
              tunnel: [Histogram_tab_reso."hist Ch 1" ("Histograms tab reso") Histogram_tab_reso."hist Ch 2" ("Histograms tab reso") Histogram_tab_reso."hist Ch 3" ("Histograms tab reso") Histogram_tab_reso."hist Ch 4" ("Histograms tab reso") Histogram_tab_reso."hist Ch 5" ("Histograms tab reso")] -> w362
              frame "Channel 1", Default {
              }
              frame "Channel 2" {
              }
              frame "Channel 3" {
              }
              frame "Channel 4" {
              }
              frame "Channel 5" {
              }
            }
            n189 = call-poly "GFGpolyGet.vi"("Variable Name in"="Histograms tab reso") -> ("output cluster"=w365:T12)  [unwired: 9 in, 1 out]
            n190 = Unbundle By Name(w365) -> ("TabControlRef"=w363:refnum<vi>)
            n191 = property class="TabCtl"(reference=w363, "Value"=w362) -> ()  [unwired: 1 in, 2 out]
          }
          frame "Objective" {
            n192 = Variant To Data(type=u16 0, Variant=w399) -> (data=w381:u16)  [unwired: 1 in, 1 out]
            n193 = Increment(x=w381) -> (x+1=w393:u16)
            n194 = Number To Decimal String(number=w393) -> (decimal integer string=w386:string)  [unwired: 1 in]
            n195 = call "GFG_core.vi"("Variable Name in"="active.objective", "Variant in"=w381, "Action"=enum16{"Init", "Set", "Get"}."Set") -> ()  [unwired: 10 in, 7 out]
            n196 = Concatenate Strings("obj", w386, ".max.field.of.view") -> (w394:string)
            n197 = Concatenate Strings("obj", w386, ".voltage.for.max.field.of.view") -> (w387:string)
            n198 = call-poly "GFGpolyGet.vi"("Variable Name in"=w394) -> ("Numeric"=w391:dbl)  [unwired: 9 in, 1 out]
            n199 = call-poly "GFGpolyGet.vi"("Variable Name in"=w387) -> ("Numeric"=w384:dbl)  [unwired: 9 in, 1 out]
            n200 = call "GFG_core.vi"("Variable Name in"="max.field.of.view", "Variant in"=w391, "Action"=enum16{"Init", "Set", "Get"}."Set") -> ()  [unwired: 10 in, 7 out]
            n201 = call "GFG_core.vi"("Variable Name in"="voltage.for.max.field.of.view", "Variant in"=w384, "Action"=enum16{"Init", "Set", "Get"}."Set") -> ()  [unwired: 10 in, 7 out]
          }
          frame "shutdown" {
          }
        }
      }
    }
    "Numeric Control 2" <- w6
  }
